vi "HostNoChopper.vi"() -> ()   [LabVIEW 2009]
uses:
  <vilib>/userDefined/High Color/nirio_resource_hc.ctl
  <instrlib>/niScope/Controls/niScope vertical coupling.ctl
  Signal Options.ctl
  Sequence.ctl
  B Field control Signal/B-Generator States.ctl
  <vilib>/Utility/error.llb/DialogType.ctl
  States.ctl
  Raman Measure/Raman.ctl
  Phase Acq.ctl
  <vilib>/DAQmx/write.llb/DAQmx Write (Analog 1D DBL 1Chan NSamp).vi
  <vilib>/DAQmx/configure/trigger.llb/DAQmx Start Trigger (Digital Edge).vi
  <vilib>/DAQmx/configure/timing.llb/DAQmx Timing (Sample Clock).vi
  <vilib>/DAQmx/create/channels.llb/DAQmx Create Channel (AO-Voltage-Basic).vi
  <vilib>/DAQmx/create/channels.llb/DAQmx Create Channel (AI-Voltage-Basic).vi
  <vilib>/DAQmx/read.llb/DAQmx Read (Analog 2D DBL NChan NSamp).vi
  <vilib>/Utility/file.llb/Write To Spreadsheet File (DBL).vi
  <vilib>/rvi/interface/nirviOpenFPGA/nirviOpenFPGA.xnode
  FPGA Bitfiles/MOT2.lvproj_FPGA Target_FPGA-no_chopper.vi.lvbitx
  FPGA-no_chopper.vi
  <vilib>/FPGAPlugInAG/Pxi-7853r/nirviIntfOpen_PXI-7853R.vi
  <vilib>/rvi/interface/nirviReadWriteControl/nirviReadWriteControl.xnode
  <vilib>/LabVIEW Targets/FPGA/Rio/nirio_HostInterface/nirio_ReadBig.vi
  <vilib>/Utility/error.llb/Error Cluster From Error Code.vi
  <vilib>/rvi/errors/niLvFpgaAdjustHostInterfaceError.vi
  <vilib>/rvi/interface/common/niFpgaNodeNameForErrorReporting.ctl
  <vilib>/rvi/errors/niLvFpgaWhatHappensToTopLevelVI.ctl
  <vilib>/RVI Host/nirviSupport.llb/nirviErrorClusterFromErrorCode.vi
  <vilib>/LabVIEW Targets/FPGA/Rio/nirio_HostInterface/nirio_WriteBig.vi
  <vilib>/rvi/interface/nirviCloseFPGA/nirviCloseFPGA.xnode
  <vilib>/FPGAPlugInAG/Pxi-7853r/nirviIntfClose_PXI-7853R.vi
  <vilib>/rvi/interface/nirviMethod/nirviMethod.xnode
  Pulse Acquisition/5122-States.ctl
  <vilib>/Analysis/NI_AALPro.lvlib
  Program Files (x86)/National Instruments/LabVIEW 2009/resource/objmgr/daqmx.rc
  <instrlib>/Agilent ESG Series/Agilent ESG Series.lvlib
  <vilib>/Analysis/NI_AALBase.lvlib
  NiRioSrv.dll
  <instrlib>/niScope/Acquire/Fetch/niScope Fetch.vi
  <instrlib>/niScope/Configure/Trigger/niScope Configure Trigger Edge.vi
  <vilib>/LabVIEW Targets/FPGA/Rio/nirio_HostInterface/nirio_DMAConfigure.vi
  <vilib>/LabVIEW Targets/FPGA/Rio/nirio_HostInterface/nirio_DMAStop.vi
panel:
  in  "Acquisition Delay":dbl[unit] format="%.2f"
  out "Interval Between Samples":dbl[unit]
  out "Actual Sample Rate":dbl[unit]
  in  "Desired Sample Rate":dbl[unit]=100000000.0 caption="Min. Sample Rate" step=1.0 format="%.2p"
  in  "Acquisition Time per Pulse":dbl[unit]=0.0005 format="%#.2g"
  out "Acquisitions Remaining":i32 caption="Number of Runs"
  in  "Number of Pulses to Record":i32=1 caption="Number of Runs" format="%.0p"
  out "Total Acquired Time":dbl[unit]
  out "Total Number of Datapoints":i32=1000000
  out "Total Experiment Time":dbl[unit]
  out "Number of Samples per Pulse":i32
  in  "Vertical range (0 to 10V)":dbl[unit]=4.0 caption="Vertical Range (V)" format="%.2f"
  in  "Vertical coupling":T1=1 caption="Vertical Coupling" items=["AC", "DC", "Ground"]
  in  "Channel":u16(ring) items=["0", "1"]
  out "Phase Frequency Pairs":dbl[][](array[numeric])
  out "Shot Noise File":path
  out "Data Directory":path
  in  "Master Stop":bool
  in  "Tab Control":T2(tab)
  out "Graphing":bool
  in  "Tab Control 3":enum32{"Timing", "TTL Signs"}(tab)
  in  "Trapping (DIO17)":dbl[unit]=0.0015 min=0.0 max=107374.18239999999
  in  "Repump (DIO18)":dbl[unit]=0.0017499999999999998
  in  "Pump (DIO19)":dbl[unit]=0.002
  in  "Memory":bool=TRUE
  in  "Shot Acquisition Trigger Duration":dbl[unit]=9.999999999999999e-06 format="%.2f"
  in  "Shot Acquisition Trigger Delay":dbl[unit] format="%.2f"
  in  "Memory Acquisition Trigger Duration":dbl[unit]=9.999999999999999e-06 format="%.2f"
  in  "Memory Acquisition Trigger Delay":dbl[unit] format="%.2f"
  in  "Acquire Shot":bool=TRUE
  in  "OD Sign":bool=TRUE
  in  "DLCZ Sign":bool=TRUE
  in  "Raman Signal Sign":bool=TRUE
  in  "Raman Control Sign":bool=TRUE
  in  "SPME Gate2 Sign":bool=TRUE
  in  "SPME Gate1 Sign":bool=TRUE
  in  "SPME Signal Sign":bool=TRUE
  in  "SPME Control Sign":bool=TRUE
  in  "Coherent Control Sign":bool
  in  "Coherent Signal Sign":bool
  in  "SQZ AOM Control Sign":bool
  in  "SQZ AOM Signal Sign":bool
  in  "SQZ AOM Signal Delay (DIO6)":dbl[unit]=0.0015
  in  "SQZ AOM Signal Duration (DIO6)":dbl[unit]=0.000125
  in  "Output  Trigger Sign (DIO13)":bool
  out "Measured Acquisition Rate":dbl[unit]=0.02 caption="Acquisition Rate" min=0.0 max=107374.18239999999
  in  "Memory Repetition Period":dbl[unit]=0.025
  out "Measured Memory Sequence Duration":dbl[unit]=0.02 min=0.0 max=107374.18239999999
  in  "DLCZ Period":dbl[unit]=1e-06
  in  "DLCZ Pulse Duration":dbl[unit]=5.0000000000000004e-08
  in  "DLCZ Stop":dbl[unit]=0.004 caption="Stop"
  in  "DLCZ Start":dbl[unit] caption="Start"
  in  "Coherent Signal Delay (DIO6)":dbl[unit]
  in  "Coherent Signal Duration (DIO6)":dbl[unit]=0.000125
  in  "Control Delay(DIO5/1)":dbl[unit] min=0.0 max=107374.18239999999
  in  "Control Duration (DIO5/1)":dbl[unit]=0.000125 min=0.0 max=107374.18239999999
  in  "FPGA Target":T3="FPGA"
  out "Active":bool
  in  "Memory Mode":T4
  out "Generated Signals":digitalwaveform(graph)
  in  "WA Extra 4 (DIO0)":dbl[unit]=0.0003
  in  "WA Extra 4 (DIO0)":dbl[unit]=2.2499999999999998e-05
  in  "WA Extra 3 (DIO0)":dbl[unit]=0.0003225
  in  "WA Extra 3 (DIO0)":dbl[unit]=2.2499999999999998e-05
  in  "WA Extra 2 (DIO0)":dbl[unit]=2.2499999999999998e-05
  in  "WA Extra 2 (DIO0)":dbl[unit]=0.0003
  in  "WA Extra (DIO0)":dbl[unit]=2.2499999999999998e-05
  in  "WA Extra  (DIO0)":dbl[unit]=0.0003225
  in  "WA Extra Sign":bool
  in  "WA Signal Switch 2  (DIO7)":dbl[unit]=0.0005269999999999997
  in  "WA Signal Switch 2 (DIO7)":dbl[unit]=8e-06
  in  "WA Signal Switch Sign":bool=TRUE
  in  "WA Signal Switch (DIO7)":dbl[unit]=0.0003169999999999997
  in  "WA Signal Switch (DIO7)":dbl[unit]=8e-06
  in  "WA Repetition Period":dbl[unit]=0.0075
  in  "WA ControlS Sign":bool=TRUE
  in  "WA Output  Trigger  Sign (DIO1)":bool
  in  "WA Signal Sign":bool
  in  "WA Repump Sign":bool
  in  "WA Pump Sign":bool
  in  "WA Control Sign":bool=TRUE
  in  "WA ControlS 2 (DIO6)":dbl[unit]=5.999999999999999e-06
  in  "WA ControlS 2 (DIO6)":dbl[unit]=0.0005249999999999996
  in  "WA Control Switch 1(DIO6)":dbl[unit]=0.00031499999999999963 min=0.0 max=107374.18239999999
  in  "WA Control Switch 1 (DIO6)":dbl[unit]=5.999999999999999e-06 min=0.0 max=107374.18239999999
  in  "WA Signal (DIO5)":dbl[unit]=2.2499999999999998e-05
  in  "WA Signal (DIO5)":dbl[unit]=0.0003
  in  "WA Repump (DIO3)":dbl[unit]=0.0007
  in  "WA Repump (DIO3)":dbl[unit]
  in  "WA Pump (DIO2)":dbl[unit]=0.0007
  in  "WA Pump (DIO2)":dbl[unit]
  in  "WA Control 2 (DIO4)":dbl[unit]=1.9999999999999998e-05
  in  "WA Control 2 (DIO4)":dbl[unit]=0.0005124999999999995
  in  "WA Control 1 (DIO4)":dbl[unit]=0.0003024999999999995 min=0.0 max=107374.18239999999
  in  "WA Control 1 (DIO4)":dbl[unit]=1.9999999999999998e-05 min=0.0 max=107374.18239999999
  out "WA Active":bool
  out "WA Reset Interval (test)":u64
  in  "Activate Raman Acquisition":bool
  in  "Scan Frequency":bool
  out "Measurement":dbl[][](graph) caption="Pulse Monitor"
  out "Raman Measure - Frequency Scan":cluster{dbl[], dbl[]}[](graph)
  in  "Ramand Control Duration (DIO5)":dbl[unit]=0.000125 min=0.0 max=107374.18239999999
  in  "Raman Control Delay(DIO5)":dbl[unit] min=0.0 max=107374.18239999999
  in  "Raman Signal Delay (DIO6)":dbl[unit]=4.9999999999999996e-05
  in  "Raman Signal Duration (DIO6)":dbl[unit]=0.000125
  in  "Linewidth":dbl[unit]=5234000.0
  in  "Detuning":dbl[unit]=10000000.0
  out "Optical Density Chart":T5(graph)
  in  "Tab Control 2":T6(tab)=enum."Threshold Settings"
  out "Optical Density Signal 2":string
  out "Optical Density Signal 1":string
  in  "OD Acquisition Delay":dbl[unit] format="%.2f"
  out "Acquisition Count":i32
  in  "Number of Measurements":u32=10
  in  "Samples per Channel":i32=2048 caption="Measurement Samples"
  out "Current Frequency":dbl[unit]
  in  "Start Frequency":dbl[unit]=-5000000.0
  in  "Stop Frequency":dbl[unit]=5000000.0
  in  "Resonance Frequency":dbl[unit]=100000000.0
  in  "Number of Frequency Intervals":u32=100
  out "Frequency Interval":dbl[unit]
  in  "Signal 2 Gain":dbl=1.0
  in  "Signal 2 Offset":dbl[unit]
  in  "Signal 1 Gain 2":dbl=1.0
  in  "Signal 1 Offset":dbl[unit]
  in  "Show Signal 2":bool
  in  "Show Reference":bool=TRUE
  in  "Show Signal 1":bool
  in  "Lower Threshold (% of Min)":dbl=110.0
  in  "Upper Threshold (% of Max)":dbl=95.0
  in  "Trigger source":tag="/Julien/PFI2"
  in  "Input Channels":tag="Julien/ai0:2"
  in  "VISA session":refnum<visa-resource-name>="GPIB0::19::INSTR"
  in  "Minimum Value":dbl[unit]=-10.0
  in  "Maximum Voltage":dbl[unit]=10.0
  in  "Acquisition Rate":dbl[unit]=5000000.0
  out "Raman Measurement File Root":path
  out "Raman Measurement File":path
  in  "Opt Density Delay (DIO7)":dbl[unit]
  in  "Opt Density Duration (DIO7)":dbl[unit]=9.999999999999999e-06
  in  "SPME Start":dbl[unit]
  in  "SPME Signal Delay(DIO5/1)":dbl[unit] min=0.0 max=107374.18239999999
  in  "SPME Signal Duration (DIO5/1)":dbl[unit]=0.000125 min=0.0 max=107374.18239999999
  in  "SPME Control Delay(DIO5/1)":dbl[unit] min=0.0 max=107374.18239999999
  in  "SPME Control Duration (DIO5/1)":dbl[unit]=0.000125 min=0.0 max=107374.18239999999
  in  "Num of SPME Pulses per Mem Seq":u64=100
  in  "SPME Period":dbl[unit]
  in  "SPME Leakage Gate Delay":dbl[unit]
  in  "SPME Leakage Gate Duration":dbl[unit]
  in  "SPME Signal Gate Delay":dbl[unit]
  in  "SPME Signal Gate Duration":dbl[unit]
  out "N1":u64
  out "N2":u64
  out "Number of Trials":u64
  in  "Desired Number of Trials":u64=100000
  in  "Tab Control 4":enum32{"Page 1", "Acquisition Settings"}(tab)=enum."Acquisition Settings"
  out "Quadrature Pulses File":path
  out "Reference Pulse File":path
  out "Acquisition Sequence":dbl[][](graph)
  in  "Get Reference Parameters":bool
  in  "Capture":bool
  in  "Acquire Data":bool
  out "Global EIT Delay":dbl[unit] format="%#.2g"
  out "Writing Phase to File":bool
  in  "Acquire Phase":bool
  in  "Physical Channel":tag="Julien/ai0,Julien/ai3"
  in  "Phase Acquisition Rate":dbl[unit]=5000000.0 caption="Sample Rate" format="%0.2f"
  in  "Minimum Value":dbl=-0.5 format="%0.2f"
  in  "Maximum Value":dbl=0.5 format="%0.2f"
  in  "samples per channel":i32=130000
  in  "Trigger Source 2":tag="/Julien/PFI1"
  out "Phase Acquisition Sampling Freq":dbl
  in  "Phase Extraction":T7(tab)=enum."Fourrier Transform Filtering Settings"
  out "Phase Monitor":dbl[][](graph)
  out "Raw Phase, Trigger, Extracted Phase Data":path
  out "Phase-Frequency Pairs":path
  out "Normalized Envelope":waveform(dbl)(graph)
  out "detected frequency":dbl format="%.4p"
  in  "Low Pass Filter Cutoff Freq: Hz":dbl=200.0
  in  "Filter Order":i32=1 min=1 max=10 step=1
  out "Memory Duration":dbl[unit]
  in  "Global Delay":dbl[unit]=3e-06
  in  "High Voltage (V Hi)":dbl[unit]=5.0
  in  "Trigger Control":bool=TRUE
  in  "Activate B-Field":bool=TRUE
  out "B-Field Control Signal":dbl[](graph)
  in  "V4":dbl[unit]
  in  "V3":dbl[unit]
  in  "V2":dbl[unit]=-5.0
  in  "V1":dbl[unit]=-5.0 min=-10.0 max=10.0
  in  "B":dbl[unit]=0.0046
  in  "A":dbl[unit]=0.0007
  in  "Trigger Source":tag="/Julien/PFI0"
  in  "Output Channel":tag="Julien/ao0"
  out "Risetime Chart":cluster{dbl}(graph)
  out "Falltime Chart":cluster{dbl}(graph)
  out "Width Chart":cluster{dbl}(graph)
  out "Delay Chart":cluster{dbl}(graph)
  out "Amplitude Chart":cluster{dbl}(graph)
  out "Risetime":string
  out "Falltime":string
  out "Pulse Width":string
  out "Delay":string
  out "Amplitude":string
  out "Current State":T8
  out "Cut Initiated":dbl[unit]
  out "Memory Mode 2":T4=enum."Coherent Memory Sequence"
  out "Memory Timer":dbl[unit]
  out "Global Time":dbl[unit]
  out "Last DLCZ Period":dbl[unit]
  out "Raman/OD Aquisition Delay":dbl[unit]
  out "Last SPME Interval Between Resets":dbl[unit]
  out "SPME Count":u64
  out "Read SPME Signal Stop":dbl[unit]
  out "Read SPME Period":dbl[unit]
  out "Read SPME Signal Start":dbl[unit]
  out "Read Num of SPME Pulses per Mem Seq":u64=100
  out "Read SPME Control Start":dbl[unit]
  out "Read SPME Control Stop":dbl[unit]
  out "Read SPME Start":dbl[unit]
  out "Memory Acquisition Trigger Delay":dbl[unit]
  out "Reference Pulse":dbl[](array[numeric])
  out "Channel String":string
  # "Delays"
  # "Durations"
  # "Coherent Signal (DIO21)"
  # "Period"
  # "Chopper Measurement and MOT Timing"
  # "Extinction Time"
  # "Alignment - Lights On"
  # "SQZ Signal (DIO23)"
  # "DLCZ Pulse Train (Signal - DIO21)"
  # "Width"
  # "Control  (DIO20)"
  # "Delays"
  # "Durations"
  # "signs"
  # "Delays"
  # "Durations"
  # "Raman Signal (DIO21)"
  # "Raman Control (DIO20"
  # "Offset"
  # "Gain"
  # "Signal 1"
  # "Signal 2"
  # "File Format:   Freq   OD1   OD2"
  # "Optical Density (DIO22)"
  # "Delay"
  # "Duration"
  # "SPME Control  (DIO20)"
  # "SPME Signal  (DIO21)"
  # "SPME Leakage Gate"
  # "SPME Signal Gate"
  # "SPME Debug"
  # "Optical Pulse Acquisition"
  # "Example Diagram"
  # "Voltages"
  # "Intervals"
  # "Trigger must be sent \nto begin generation"
  # "Pulse Statistics"
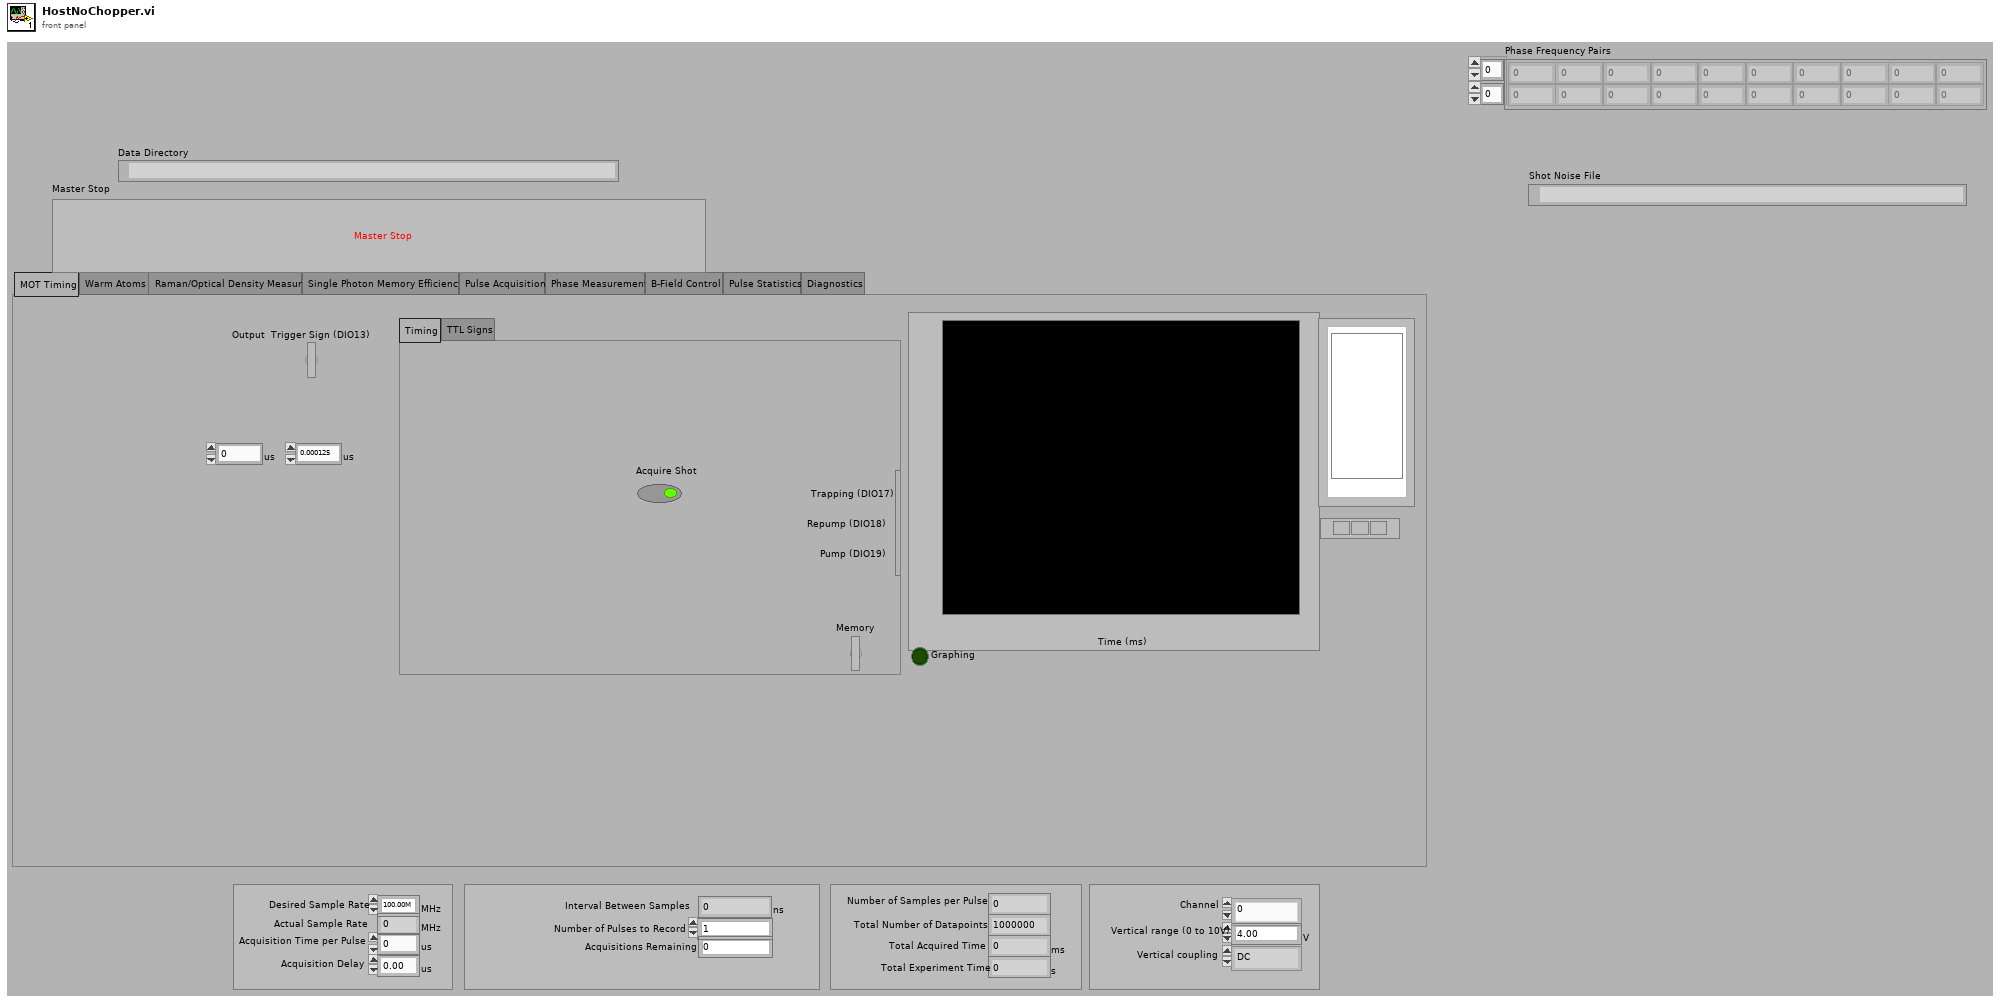
[diagram p1: front panel]
types:
  T1 = typedef "niScope vertical coupling.ctl" = i32
  T2 = enum32{"MOT Timing", "Warm Atoms", "Raman/Optical Density Measure", "Single Photon Memory Efficiency", "Pulse Acquisition", "Phase Measurement", "B-Field Control", "Pulse Statistics", "Diagnostics"}
  T3 = typedef "nirio_resource_hc.ctl" = tag
  T4 = typedef "Signal Options.ctl" = enum16{"Cycle Trap - Standby", "Generate DLCZ Pulses", "Measure Optical Density", "Measure Raman", "Single Photon Memory Efficiency", "Coherent Memory Sequence", "Squeezed AOM Memory Sequence", "Squeezed Chopper Memory Sequence"}
  T5 = cluster{"Optical Density 1":dbl, "Optical Density 2":dbl}
  T6 = enum32{"Parameters", "Threshold Settings", "Acquisition Settings"}
  T7 = enum32{"Arches and Phase Monitor", "Fourrier Transform Filtering Settings"}
  T8 = typedef "Sequence.ctl" = enum16{"Build MOT", "Memory Sequence", "Alignment - Lights On"}
  T9 = enum16{"open", "replace", "create", "open or create", "replace or create", "replace or create with confirmation"}
  T10 = typedef "Phase Acq.ctl" = enum16{"Start Phase Acquisition", "Monitor Phase", "Stop Phase Acquisition", "Restart", "Standby"}
  T11 = typedef "Raman.ctl" = enum16{"Initialize", "Monitor Pulses", "Stop Raman Acquisition", "Scan Frequency", "Output Data", "Standby"}
  T12 = typedef "States.ctl" = enum16{"Initialize", "Send Data", "Receive Data", "Update Graph", "Check for Activity", "Close"}
  T13 = typedef "DialogType.ctl" = u16
  T14 = typedef "B-Generator States.ctl" = enum16{"Initialize", "Start Task", "Check Task", "Stop Task", "Stop"}
  T15 = typedef "5122-States.ctl" = enum16{"Initialize Card", "Continuous Mode", "Fetch", "Snapshot Acquistion", "Standby", "Record DataFile", "Exit"}
  T16 = cluster{"Optical Density 1":dbl, "Optical Density 2":dbl}[]
  T17 = cluster{"Phase Acquisition Sampling Freq":dbl, "samples per channel":i32}
  T18 = typedef "niFpgaNodeNameForErrorReporting.ctl" = enum16{"Open FPGA VI Reference", "Read/Write Control", "Invoke Method: Abort", "Invoke Method: Acknowledge IRQ", "Invoke Method: Download", "Invoke Method: FIFO.Configure", "Invoke Method: FIFO.Read", "Invoke Method: FIFO.Start", "Invoke Method: FIFO.Stop", "Invoke Method: FIFO.Write", "Invoke Method: Reset", "Invoke Method: Run", "Invoke Method: Wait on IRQ", "Close FPGA VI Reference"}
  T19 = typedef "niLvFpgaWhatHappensToTopLevelVI.ctl" = enum16{"top level VI scripted behind XNode", "top level VI inlined behind XNode"}
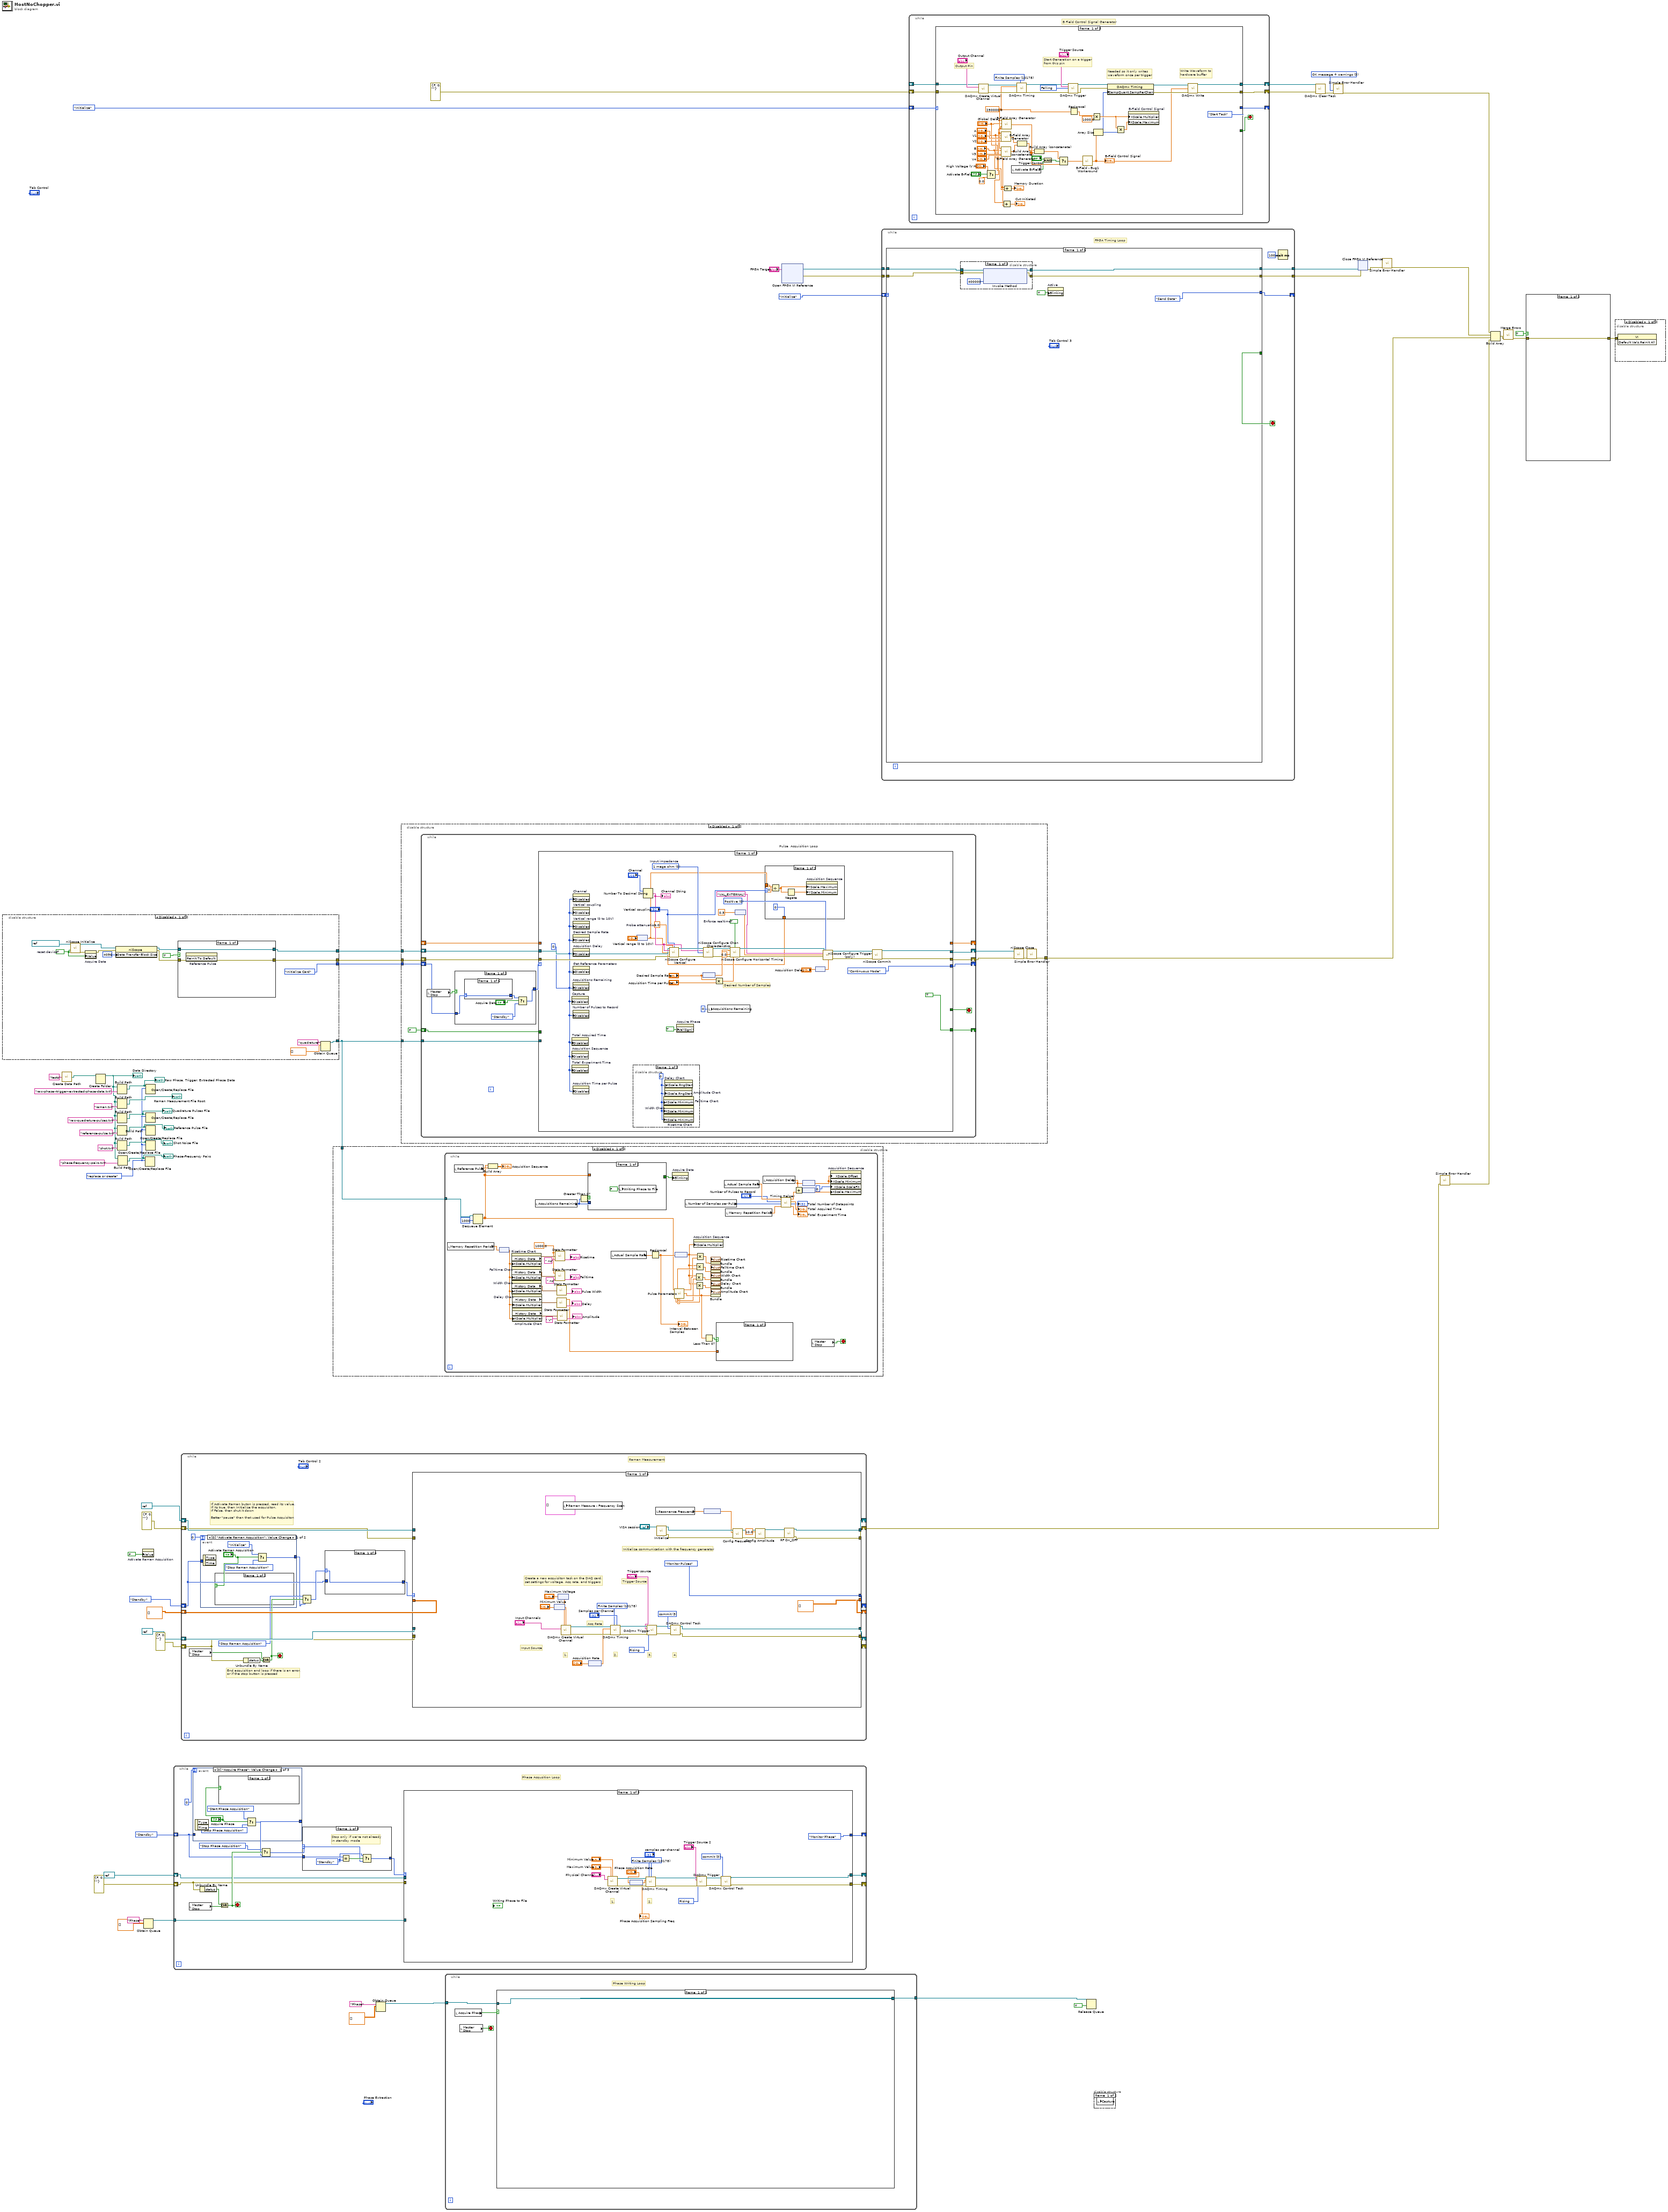
[diagram p0: block diagram]
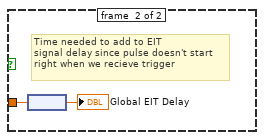
[diagram p2: hidden frame]
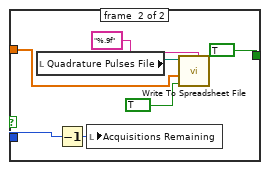
[diagram p3: hidden frame]
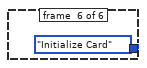
[diagram p9: hidden frame]
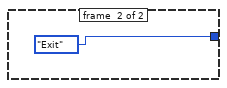
[diagram p10: hidden frame]
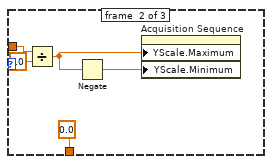
[diagram p12: hidden frame]
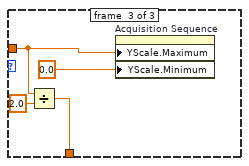
[diagram p13: hidden frame]
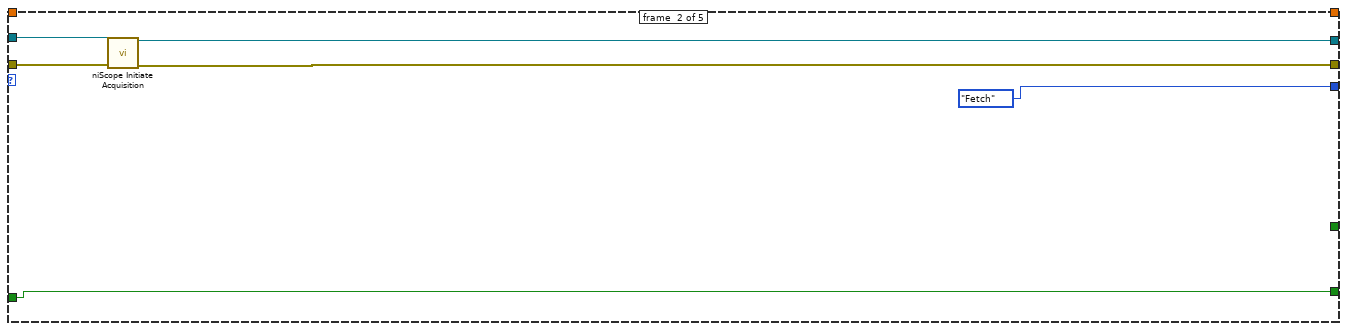
[diagram p14: hidden frame]
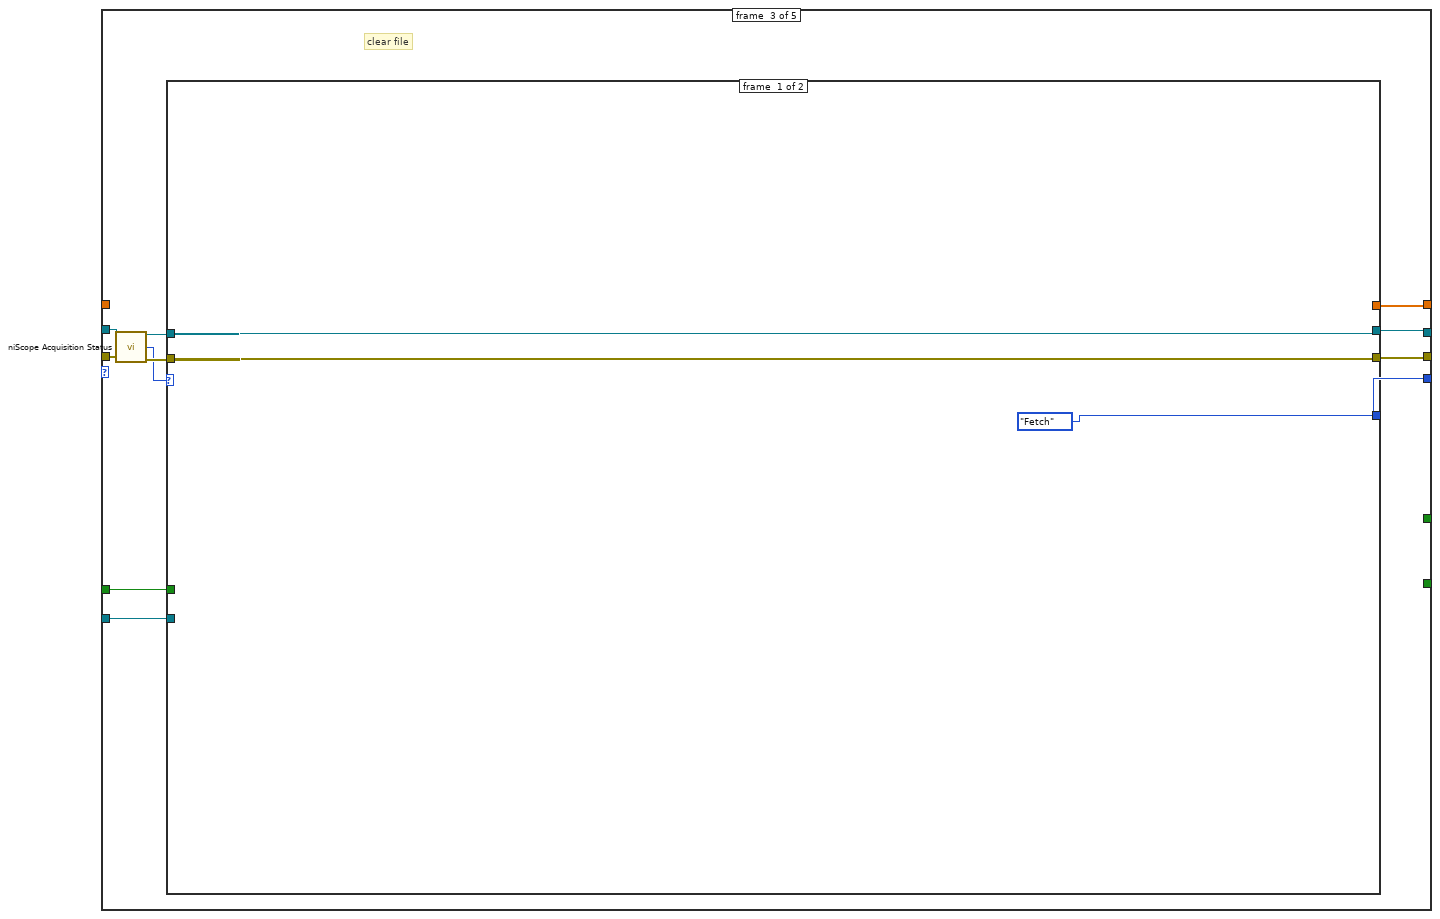
[diagram p15: hidden frame]
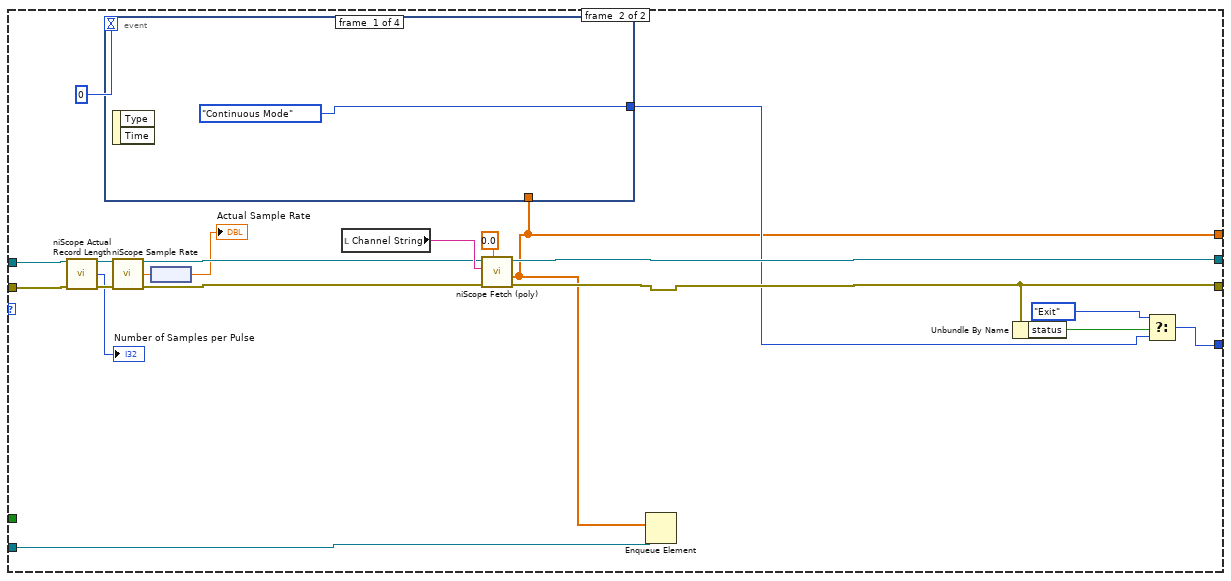
[diagram p16: hidden frame]
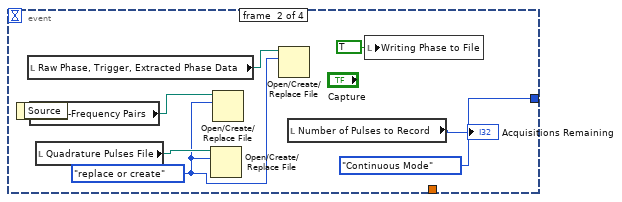
[diagram p17: hidden frame]
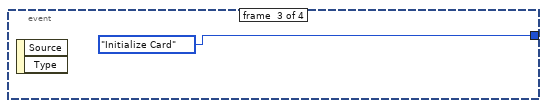
[diagram p18: hidden frame]
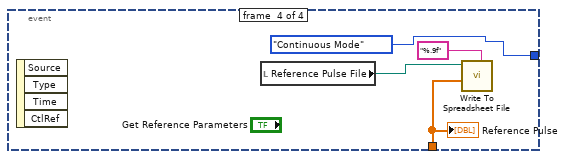
[diagram p19: hidden frame]
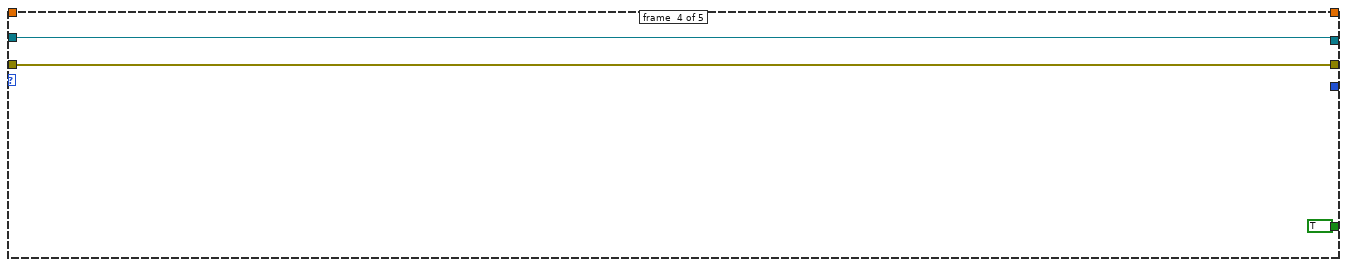
[diagram p20: hidden frame]
diagram:
  w2 = T9."replace or create" ("operation (0:open)")
  w57 = T13 3 items=["no dialog", "OK message", "continue or stop message", "OK message + warnings", "continue/stop + warnings"] ("type of dialog (OK msg:1)")
  n1 = disable-structure shown="Disabled" {
    disable-tunnel: [w67 _] -> w60
    disable-tunnel: [w65 _] -> w59
    disable-tunnel: [5122-States."Initialize Card" ("Enum") _] -> w58
    disable-tunnel: [w61 _] -> w1
    frame #0 {
      w70 = TRUE  # reset device
      n2 = call <instrlib>:"niScope Initialize.vi"("resource name"=refnum<k15> "Acquisition" ("Resource name 5"), "reset device"=w70) -> ("instrument handle"=w74:refnum<k15>, "error out"=w72:errorcluster)  [unwired: 2 in, 10 out]
      n3 = property on="Acquire Data" class="Bool (strict)"(error in=w72, "Value"=w70) -> (error out=w71:errorcluster)  [unwired: 1 in, 1 out]
      n4 = property class="niScope"(reference=w74, error in=w71, "Data Transfer Block Size"=4096) -> (reference out=w68:refnum<k15>, error out=w66:errorcluster)
      n5 = case shown="True" TRUE {
        tunnel: [w77 w79] -> w67
        tunnel: w68 -> [w77 w79]
        tunnel: [w76 w78] -> w65
        tunnel: w66 -> [w76 w78]
        frame #0 {
          n6 = invoke on="Reference Pulse" class="Arr (strict)" method="Reinit To Default"() -> ()  [unwired: 3 in, 3 out]
        }
        frame #1 {
        }
      }
      n7 = Obtain Queue(name (unnamed)="quadrature", element data type=dbl[] [] ("wfm")) -> (queue out=w61:refnum<queue>)  [unwired: 3 in, 2 out]
    }
    frame #1 {
    }
  }
  n8 = call "Create Data Path.vi"("Data Directory Name"="tests") -> ("appended path"=w13:path)
  n9 = Create Folder(path (use dialog)=w13) -> (created path=w4:path)  [unwired: 2 in, 2 out]
  "Data Directory" <- w4
  n10 = Build Path(base path=w4, name or relative path="raw-phase--trigger--extracted-phase-data.txt") -> (appended path=w11:path)
  "Raw Phase, Trigger, Extracted Phase Data" <- w11
  n11 = Build Path(base path=w4, name or relative path="raman.txt") -> (appended path=→"Raman Measurement File Root":path)
  n12 = Build Path(base path=w4, name or relative path="raw-quadrature-pulses.txt") -> (appended path=w9:path)
  "Quadrature Pulses File" <- w9
  n13 = Build Path(base path=w4, name or relative path="reference-pulse.txt") -> (appended path=w8:path)
  "Reference Pulse File" <- w8
  n14 = Build Path(base path=w4, name or relative path="shot.txt") -> (appended path=w7:path)
  "Shot Noise File" <- w7
  n15 = Build Path(base path=w4, name or relative path="phase-frequency-pairs.txt") -> (appended path=w3:path)
  "Phase-Frequency Pairs" <- w3
  n16 = property on="Activate Raman Acquisition" class="Bool (strict)"("Value"=FALSE ("Activate Raman Acquisition")) -> ()  [unwired: 2 in, 2 out]
  n17 = Obtain Queue(name (unnamed)="Phase", element data type=dbl[][] [] ("data")) -> (queue out=w22:refnum<queue>)  [unwired: 3 in, 2 out]
  n18 = Open/Create/Replace File(file path (use dialog)=w3, operation (0:open)=w2) -> ()  [unwired: 4 in, 3 out]
  n19 = Open/Create/Replace File(file path (use dialog)=w11, operation (0:open)=w2) -> ()  [unwired: 4 in, 3 out]
  n20 = Open/Create/Replace File(file path (use dialog)=w9, operation (0:open)=w2) -> ()  [unwired: 4 in, 3 out]
  n21 = Open/Create/Replace File(file path (use dialog)=w8, operation (0:open)=w2) -> ()  [unwired: 4 in, 3 out]
  n22 = Open/Create/Replace File(file path (use dialog)=w7, operation (0:open)=w2) -> ()  [unwired: 4 in, 3 out]
  n23 = while {
    shift-right: [w86] -> _
    shift-left: refnum<k21> refnum ("task out") -> [w84]
    shift-right: [w85] -> _
    shift-left: errorcluster {"status"=FALSE, "code"=0, "source"=""} ("error out") -> [w82]
    shift-right: [w83] -> _
    shift-left: Phase_Acq."Standby" ("Enum") -> [w88]
    tunnel: w22 -> [w80]
    stop <- w91 stop-if-true
    # "Phase Acqusition Loop"
    n24 = local read "Master Stop"() -> (w93:bool)
    n25 = event shown="[0] \"Acquire Phase\": Value Change" {
      selector: _ -> [_ _ _]
      dyn-events: _ -> [_ _ _]
      timeout: 0 -> [_ _ _]
      tunnel: [w158 Phase_Acq."Restart" ("Enum") w161] -> w90
      tunnel: w88 -> [_ _ w161]
      event #0 {
        n26 = event-data() -> ()  [unwired: 1 in, 2 out]
        n27 = case shown="True" "Acquire Phase" {
          frame #0 {
          }
          frame #1 {
            # "Disabled Raman Acquisiton if we want to start\nPhase Acq.  Uses same cards"
            n28 = property on="Activate Raman Acquisition" class="Bool (strict)"("Val(Sgnl)"=FALSE ("Value (Signaling)")) -> ()  [unwired: 2 in, 2 out]
          }
        }
        n29 = Select(t=Phase_Acq."Start Phase Acquisition" ("Enum"), s="Acquire Phase", f=Phase_Acq."Stop Phase Acquisition" ("Enum")) -> (s? t:f=w158:T10)
      }
      event #1 {
        n30 = event-data() -> ()  [unwired: 1 in, 3 out]
      }
      event #2 {
        n31 = event-data() -> ()  [unwired: 1 in, 2 out]
      }
    }
    n32 = Unbundle By Name(w82) -> ("status"=w81:bool)
    n33 = Or(x=w81, y=w93) -> (x .or. y?=w91:bool)
    n34 = Select(t=Phase_Acq."Stop Phase Acquisition" ("Enum"), s=w91, f=w90) -> (s? t:f=w92:T10)
    n35 = case shown="\"Standby\"" w92 {
      selector: w92 -> [w148 w151 w152 w153 w154]
      tunnel: w88 -> [w150 _ _ _ _]
      tunnel: [w147 w151 w152 w153 w154] -> w87
      frame #0 {
        w146 = Phase_Acq."Standby" ("Enum")
        # "Stop only if we're not already\nin standby mode"
        n36 = Equal?(x=w150, y=w146) -> (x = y?=w149:bool)
        n37 = Select(t=w146, s=w149, f=w148) -> (s? t:f=w147:T10)
      }
      frame #1 {
      }
      frame #2 {
      }
      frame #3 {
      }
      frame #4 {
      }
    }
    n38 = case shown="\"Restart\"" w87 {
      tunnel: [w98 refnum<k21> refnum ("task out") refnum<k21> refnum ("task out") refnum<k21> refnum ("task out") w145] -> w86
      tunnel: [w97 errorcluster {"status"=FALSE, "code"=0, "source"=""} ("error out") errorcluster {"status"=FALSE, "code"=0, "source"=""} ("error out") errorcluster {"status"=FALSE, "code"=0, "source"=""} ("error out") w144] -> w85
      tunnel: w84 -> [_ w118 w125 _ w143]
      tunnel: w82 -> [_ w117 w124 _ w142]
      tunnel: [Phase_Acq."Monitor Phase" ("Enum") Phase_Acq."Standby" ("Enum") Phase_Acq."Start Phase Acquisition" ("Enum") Phase_Acq."Standby" ("Enum") Phase_Acq."Monitor Phase" ("Enum")] -> w83
      tunnel: w80 -> [_ _ _ _ w131]
      frame #0 {
        w99 = 3 items=["verify"=2, "reserve"=4, "commit"=3, "unreserve"=5, "abort"=6] ("action")
        w103 = 10280 items=["Rising"=10280, "Falling"=10171] ("edge")
        w113 = 10178 items=["Finite Samples"=10178, "Continuous Samples"=10123] ("sample mode")
        # "2."
        # "1."
        n39 = call-poly <vilib>:"DAQmx Create Virtual Channel.vi"("maximum value"="Maximum Value", "minimum value"="Minimum Value", "physical channels"="Physical Channel") -> ("task out"=w111:refnum<k21>, "error out"=w110:errorcluster)  [unwired: 6 in, 5 out]
        n40 = node("Phase Acquisition Rate") -> (w95:dbl)
        "Phase Acquisition Sampling Freq" <- w95
        n41 = call-poly <vilib>:"DAQmx Timing.vi"("task/channels in"=w111, "sample mode"=w113, "samples per channel"="samples per channel", "rate"=w95, "error in"=w110) -> ("task out"=w105:refnum<k21>, "error out"=w104:errorcluster)  [unwired: 2 in, 7 out]
        n42 = call-poly <vilib>:"DAQmx Trigger.vi"("task/channels in"=w105, "source"="Trigger Source 2", "edge"=w103, "error in"=w104) -> ("task out"=w101:refnum<k21>, "error out"=w100:errorcluster)  [unwired: 10 in]
        n43 = call <vilib>:"DAQmx Control Task.vi"("task/channels in"=w101, "action"=w99, "error in"=w100) -> ("task out"=w98:refnum<k21>, "error out"=w97:errorcluster)  [unwired: 11 in]
      }
      frame #1 {
        w120 = T13 3 items=["no dialog", "OK message", "continue or stop message", "OK message + warnings", "continue/stop + warnings"] ("type of dialog (OK msg:1)")
        n44 = call <vilib>:"DAQmx Clear Task.vi"("task in"=w118, "error in"=w117) -> ("error out"=w119:errorcluster)  [unwired: 13 out]
        n45 = call <vilib>:"Simple Error Handler.vi"("type of dialog (OK msg:1)"=w120, "error in (no error)"=w119) -> ()  [unwired: 8 out]
      }
      frame #2 {
        w127 = T13 3 items=["no dialog", "OK message", "continue or stop message", "OK message + warnings", "continue/stop + warnings"] ("type of dialog (OK msg:1)")
        n46 = call <vilib>:"DAQmx Clear Task.vi"("task in"=w125, "error in"=w124) -> ("error out"=w126:errorcluster)  [unwired: 13 out]
        n47 = call <vilib>:"Simple Error Handler.vi"("type of dialog (OK msg:1)"=w127, "error in (no error)"=w126) -> ()  [unwired: 8 out]
      }
      frame #3 {
      }
      frame #4 {
        w133 = u8 0 ("X Scale.Scale Fit")
        # "4."
        n48 = local read "Phase Acquisition Rate"() -> (w140:dbl[unit])
        n49 = local read "samples per channel"() -> (w137:i32)
        n50 = node(w140) -> (w139:dbl)
        n51 = Reciprocal(x=w139) -> (1/x=w136:dbl)
        n52 = Multiply(x=w137, y=w136) -> (x*y=w135:dbl)
        n53 = Add(x=w133, y=w135) -> (x+y=w134:dbl)
        n54 = property on="Phase Monitor" class="WFGraph (strict)"("XScale.Offset"=w133, "XScale.Minimum"=w133, "XScale.Maximum"=w134, "XScale.ScaleFit"=u8 0 ("X Scale.Scale Fit"), "XScale.Multiplier"=w136) -> ()  [unwired: 2 in, 2 out]
        n55 = call-poly <vilib>:"DAQmx Read.vi"("task/channels in"=w143, "error in"=w142) -> ("task out"=w145:refnum<k21>, "data"=w132:dbl[][], "error out"=w144:errorcluster)  [unwired: 2 in, 9 out]
        n56 = Enqueue Element(queue=w131, element=w132) -> ()  [unwired: 2 in, 3 out]
      }
    }
  }
  n57 = while {
    shift-right: [w177] -> _
    shift-left: Raman."Standby" ("Raman State") -> [w163]
    shift-right: [w180] -> _
    shift-left: refnum<k21> refnum ("task out") -> [w176]
    shift-right: [w181] -> _
    shift-left: errorcluster {"status"=FALSE, "code"=0, "source"=""} ("error out") -> [w171]
    shift-right: [w172] -> _
    shift-left: dbl[][] [] -> [w175]
    shift-right: [w178] -> _
    shift-left: refnum<visa-resource-name> refnum ("VISA Resource Name Out") -> [w174]
    shift-right: [w179] -> w36
    shift-left: errorcluster {"status"=FALSE, "code"=0, "source"=""} ("error out") -> [w173]
    stop <- w167 stop-if-true
    # "If Activate Raman buton is pressed, read its value.\nIf its true, then Initialize the acquisiton, \nIf False, then shut it down\n\nBetter \"pause\" than that used for Pulse Acquisiton"
    # "End acquisition and loop if there is an error, \nor if the stop button is pressed"
    # "Raman Measurement"
    n58 = local read "Master Stop"() -> (w169:bool)
    n59 = event shown="[0] \"Activate Raman Acquisition\": Value Change" {
      selector: _ -> [_ _]
      dyn-events: _ -> [_ _]
      timeout: 0 -> [_ _]
      tunnel: [w193 w197] -> w165
      tunnel: w163 -> [_ w197]
      event #0 {
        n60 = event-data() -> ()  [unwired: 1 in, 2 out]
        n61 = case shown="True" "Activate Raman Acquisition" {
          frame #0 {
          }
          frame #1 {
            # "Disabled Phase Acquisiton if we want to start\nRaman Acq.  Uses same cards"
            n62 = property on="Acquire Phase" class="Bool (strict)"("Val(Sgnl)"=FALSE ("Value (Signaling)")) -> ()  [unwired: 2 in, 2 out]
          }
        }
        n63 = Select(t=Raman."Initialize" ("Raman State"), s="Activate Raman Acquisition", f=Raman."Stop Raman Acquisition" ("Raman State")) -> (s? t:f=w193:T11)
      }
      event #1 {
        n64 = event-data() -> ()  [unwired: 1 in, 2 out]
      }
    }
    n65 = Unbundle By Name(w171) -> ("status"=w170:bool)
    n66 = Or(x=w169, y=w170) -> (x .or. y?=w167:bool)
    n67 = Select(t=Raman."Stop Raman Acquisition" ("Raman State"), s=w167, f=w165) -> (s? t:f=w164:T11)
    n68 = case shown="\"Standby\"" w164 {
      selector: w164 -> [w182 w183 w185 w189 w190 w191]
      tunnel: w163 -> [_ _ w188 _ _ _]
      tunnel: [w182 w183 w184 w189 w190 w191] -> w162
      frame #0 {
      }
      frame #1 {
      }
      frame #2 {
        w186 = Raman."Standby" ("Raman State")
        # "Stop only if we're not already\nin standby mode"
        n69 = Equal?(x=w188, y=w186) -> (x = y?=w187:bool)
        n70 = Select(t=w186, s=w187, f=w185) -> (s? t:f=w184:T11)
      }
      frame #3 {
      }
      frame #4 {
      }
      frame #5 {
      }
    }
    n71 = case shown="\"Monitor Pulses\"" w162 {
      tunnel: [w216 w272 w308 w359 errorcluster {"status"=FALSE, "code"=0, "source"=""} ("error out") w382] -> w181
      tunnel: [w217 w273 w307 w360 refnum<k21> refnum ("task out") refnum<k21> refnum ("task out")] -> w180
      tunnel: [w204 w277 w293 w357 w368 errorcluster {"status"=FALSE, "code"=0, "source"=""} ("error out")] -> w179
      tunnel: [w203 w278 w294 w358 w369 refnum<visa-resource-name> refnum ("VISA Resource Name Out")] -> w178
      tunnel: [Raman."Monitor Pulses" ("Raman State") w271 Raman."Output Data" ("Raman State") Raman."Monitor Pulses" ("Raman State") Raman."Standby" ("Raman State") Raman."Standby" ("Raman State")] -> w177
      tunnel: w176 -> [_ w275 w300 w360 _ w384]
      tunnel: w171 -> [_ w274 w299 w359 _ w383]
      tunnel: w175 -> [_ _ _ w362 _ _]
      tunnel: w174 -> [_ w278 w297 w358 w369 w372]
      tunnel: w173 -> [_ w277 w296 w357 w368 w371]
      tunnel: [dbl[][] [] ("Frequency/Delta Pairs") _ w284 _ _ _] -> w172
      frame #0 {
        w232 = 10280 items=["Rising"=10280, "Falling"=10171] ("edge")
        w223 = 3 items=["verify"=2, "reserve"=4, "commit"=3, "unreserve"=5, "abort"=6] ("action")
        w224 = 10178 items=["Finite Samples"=10178, "Continuous Samples"=10123] ("sample mode")
        # "Initialize communication with the frequency generator"
        # "Create a new acquisiton task on the DAQ card, \nset settings for voltage, Acq rate, and triggers"
        # "Input Source"
        # "Acq Rate"
        # "Trigger Source"
        # "4."
        # "3."
        # "2."
        # "1."
        n72 = node("Minimum Value") -> (w198:dbl)
        n73 = node("Maximum Voltage") -> (w199:dbl)
        n74 = call-poly <vilib>:"DAQmx Create Virtual Channel.vi"("maximum value"=w199, "minimum value"=w198, "physical channels"="Input Channels") -> ("task out"=w226:refnum<k21>, "error out"=w229:errorcluster)  [unwired: 11 in]
        n75 = local write "Raman Measure - Frequency Scan"(cluster{dbl[], dbl[]}[] [] ("Raman Measure")) -> ()
        n76 = node("Acquisition Rate") -> (w200:dbl)
        n77 = call-poly <vilib>:"DAQmx Timing.vi"("task/channels in"=w226, "sample mode"=w224, "samples per channel"="Samples per Channel", "rate"=w200, "error in"=w229) -> ("task out"=w222:refnum<k21>, "error out"=w221:errorcluster)  [unwired: 9 in]
        n78 = call-poly <vilib>:"DAQmx Trigger.vi"("task/channels in"=w222, "source"="Trigger source", "edge"=w232, "error in"=w221) -> ("task out"=w220:refnum<k21>, "error out"=w219:errorcluster)  [unwired: 10 in]
        n79 = local read "Resonance Frequency"() -> (w211:dbl[unit])
        n80 = call <instrlib>:"Initialize.vi"("VISA Resource Name"="VISA session") -> ("VISA Resource Name Out"=w213:refnum<visa-resource-name>, "error out"=w212:errorcluster)  [unwired: 4 in, 9 out]
        n81 = call <vilib>:"DAQmx Control Task.vi"("task/channels in"=w220, "action"=w223, "error in"=w219) -> ("task out"=w217:refnum<k21>, "error out"=w216:errorcluster)  [unwired: 11 in]
        n82 = node(w211) -> (w210:dbl)
        n83 = call <instrlib>:"Config Frequency.vi"("VISA Resource Name"=w213, "Frequency (1000.0)"=w210, "error in (no error)"=w212) -> ("VISA Resource Name Out"=w209:refnum<visa-resource-name>, "error out"=w208:errorcluster)  [unwired: 6 in, 5 out]
        n84 = call <instrlib>:"Config Amplitude.vi"("VISA Resource Name"=w209, "Amplitude (-135.00)"=10.0, "error in (no error)"=w208) -> ("VISA Resource Name Out"=w206:refnum<visa-resource-name>, "error out"=w205:errorcluster)  [unwired: 5 in, 6 out]
        n85 = call <instrlib>:"RF On_OFF.vi"("VISA Resource Name"=w206, "error in (no error)"=w205) -> ("VISA Resource Name Out"=w203:refnum<visa-resource-name>, "error out"=w204:errorcluster)  [unwired: 1 in, 11 out]
      }
      frame #1 {
        n86 = local read "Acquisition Rate"() -> (w258:dbl[unit])
        n87 = local read "OD Acquisition Delay"() -> (w257:dbl[unit])
        n88 = local read "Samples per Channel"() -> (w259:i32)
        n89 = node(w258) -> (w256:dbl)
        n90 = Reciprocal(x=w256) -> (1/x=w253:dbl)
        n91 = node(w257) -> (w255:dbl)
        n92 = Multiply(x=w259, y=w253) -> (x*y=w254:dbl)
        n93 = Add(x=w255, y=w254) -> (x+y=w252:dbl)
        n94 = property on="Measurement" class="WFGraph (strict)"("XScale.Offset"=w255, "XScale.Minimum"=w255, "XScale.Maximum"=w252, "XScale.ScaleFit"=u8 0 ("X Scale.Scale Fit"), "XScale.Multiplier"=w253) -> ()  [unwired: 2 in, 2 out]
        n95 = call-poly <vilib>:"DAQmx Read.vi"("task/channels in"=w275, "error in"=w274) -> ("task out"=w273:refnum<k21>, "data"=w240:dbl[][], "error out"=w272:errorcluster)  [unwired: 11 in]
        n96 = property on="Optical Density Chart" class="WFChart (strict)"() -> ("History Data"=w265:T16)  [unwired: 2 in, 2 out]
        n97 = call "OD Stats Formatter.vi"("OD History"=w265) -> ("Statistics String"=→"Optical Density Signal 1":string, "Statistics String 2"=→"Optical Density Signal 2":string)  [unwired: 9 in, 4 out]
        n98 = call "Numerical Offset and Gain.vi"("Signal 1 Offset"="Signal 1 Offset", "Signal 2 Offset"="Signal 2 Offset", "Signal 1 Gain"="Signal 1 Gain 2", "Signal 2 Gain"="Signal 2 Gain", "Input Data"=w240) -> ("Output Data"=w235:dbl[][])
        n99 = local read "Samples per Channel"() -> (w242:i32)
        n100 = call "2-Ch Optical Density.vi"("Detuning"="Detuning", "Linewidth"="Linewidth", "data"=w235, "Upper Threshold (% of Max)"="Upper Threshold (% of Max)", "Lower Threshold (% of Min)"="Lower Threshold (% of Min)") -> ("Upper Voltage Threshold Reference"=w251:dbl, "Upper Voltage Threshold Signal 1"=w248:dbl, "Upper Voltage Threshold Signal 2"=w244:dbl, "Optical Density 1"=w268:dbl, "Lower Voltage Threshold Reference"=w250:dbl, "Lower Voltage Threshold Signal 1"=w247:dbl, "Lower Voltage Threshold Signal 2"=w245:dbl, "Optical Density 2"=w267:dbl)  [unwired: 3 in]
        n101 = call "Group Reference Toggle.vi"("Samples per Channel"=w242, "Show Reference"="Show Reference", "Show Signal 1"="Show Signal 1", "Show Signal 2"="Show Signal 2", "Upper Voltage Threshold Reference"=w251, "Upper Voltage Threshold Signal 1"=w248, "Lower Voltage Threshold Reference"=w250, "Upper Voltage Threshold Signal 2"=w244, "Lower Voltage Threshold Signal 1"=w247, "Lower Voltage Threshold Signal 2"=w245) -> ("Array"=w241:dbl[][])  [unwired: 2 in, 3 out]
        n102 = Bundle("Optical Density 1"=w268, "Optical Density 2"=w267) -> (→"Optical Density Chart":T5)  [unwired: 1 in]
        n103 = event shown="[1] \"Scan Frequency\": Value Change" {
          selector: _ -> [_ _]
          dyn-events: _ -> [_ _]
          timeout: 0 -> [_ _]
          tunnel: [Raman."Monitor Pulses" ("Raman State") Raman."Scan Frequency" ("Raman State")] -> w271
          event #0 {
            n104 = event-data() -> ()  [unwired: 1 in, 2 out]
          }
          event #1 {
            n105 = event-data() -> ()  [unwired: 1 in, 5 out]
          }
        }
        n106 = Build Array (concatenate)(w235, w241) -> (w234:dbl[][])
        n107 = call "-1 V Offset.vi"("Input Data"=w234) -> ("Output Data"=→"Measurement":dbl[][])
      }
      frame #2 {
        n108 = call "Convert Frequencies.vi"("Resonance Frequency (MHz)"="Resonance Frequency", "Number of Intervals"="Number of Frequency Intervals", "Start Frequency (MHz)"="Start Frequency", "Stop Frequency (MHz)"="Stop Frequency") -> ("Start Frequency (Number)"=w302:dbl, "Frequency Increment (Number)"=w303:dbl, "Number of Intervals (Out)"=w304:u32, "Frequency Interval"=→"Frequency Interval":dbl[unit])
        n109 = for {
          N: w304 -> [_]
          shift-right: [w330] -> w307
          shift-left: w300 -> [w328]
          shift-right: [w331] -> w308
          shift-left: w299 -> [w329]
          tunnel: w303 -> [w325]
          shift-right: [w320] -> _
          shift-left: w302 -> [w312]
          shift-right: [w322] -> w295
          shift-left: w297 -> [w324]
          shift-right: [w321] -> w292
          shift-left: w296 -> [w323]
          tunnel: [w310] -> w285 mode=indexing
          tunnel: [w309] -> w282 mode=indexing
          tunnel: [w315] -> w281 mode=indexing
          n110 = for {
            N: "Number of Measurements" -> [_]
            shift-right: [w344] -> w330
            shift-left: w328 -> [w346]
            shift-right: [w343] -> w331
            shift-left: w329 -> [w345]
            tunnel: [w349] -> w326 mode=indexing
            tunnel: [w348] -> w316 mode=indexing
            i -> [w350]
            stop <- w351 stop-if-true
            w353 = 10.0  # timeout
            # "Acquisition Block"
            # "Send reference into AI0 and Signal into AI1 and AI2"
            n111 = local read "Lower Threshold (% of Min)"() -> (w339:dbl)
            n112 = local read "Upper Threshold (% of Max)"() -> (w340:dbl)
            n113 = local read "Signal 1 Gain 2"() -> (w335:dbl)
            n114 = local read "Signal 1 Offset"() -> (w337:dbl[unit])
            n115 = local read "Signal 2 Offset"() -> (w336:dbl[unit])
            n116 = local read "Linewidth"() -> (w341:dbl[unit])
            n117 = local read "Detuning"() -> (w342:dbl[unit])
            n118 = local read "Signal 2 Gain"() -> (w334:dbl)
            n119 = call-poly <vilib>:"DAQmx Read.vi"("task/channels in"=w346, "timeout"=w353, "error in"=w345) -> ("task out"=w344:refnum<k21>, "data"=w338:dbl[][], "error out"=w343:errorcluster)  [unwired: 10 in]
            n120 = call "Numerical Offset and Gain.vi"("Signal 1 Offset"=w337, "Signal 2 Offset"=w336, "Signal 1 Gain"=w335, "Signal 2 Gain"=w334, "Input Data"=w338) -> ("Output Data"=w333:dbl[][])
            n121 = call "2-Ch Optical Density.vi"("Detuning"=w342, "Linewidth"=w341, "data"=w333, "Upper Threshold (% of Max)"=w340, "Lower Threshold (% of Min)"=w339) -> ("Optical Density 1"=w349:dbl, "Optical Density 2"=w348:dbl)  [unwired: 3 in, 6 out]
            n122 = Unbundle By Name(w343) -> ("status"=w352:bool)
            n123 = call "-1 V Offset.vi"("Input Data"=w333) -> ("Output Data"=w332:dbl[][])
            n124 = local write "Measurement"(w332) -> ()
            n125 = Or(x=w352, y=FALSE) -> (x .or. y?=w351:bool)
            "Acquisition Count" <- w350
          }
          n126 = call <instrlib>:"Config Frequency.vi"("VISA Resource Name"=w324, "Frequency (1000.0)"=w312, "error in (no error)"=w323) -> ("VISA Resource Name Out"=w318:refnum<visa-resource-name>, "error out"=w319:errorcluster)  [unwired: 6 in, 5 out]
          n127 = node(w312) -> (→"Current Frequency":dbl[unit])
          n128 = Add(x=w325, y=w312) -> (x+y=w320:dbl)
          n129 = local read "Resonance Frequency"() -> (w314:dbl[unit])
          n130 = call <instrlib>:"Config Amplitude.vi"("VISA Resource Name"=w318, "Amplitude (-135.00)"=10.0, "error in (no error)"=w319) -> ("VISA Resource Name Out"=w322:refnum<visa-resource-name>, "error out"=w321:errorcluster)  [unwired: 5 in, 6 out]
          n131 = node(w314) -> (w313:dbl)
          n132 = Subtract(x=w312, y=w313) -> (x-y=w309:dbl)
          n133 = call <vilib>:"Std Deviation and Variance.vi"("X"=w326) -> ("mean"=w310:dbl)  [unwired: 1 in, 2 out]
          n134 = call <vilib>:"Std Deviation and Variance.vi"("X"=w316) -> ("mean"=w315:dbl)  [unwired: 1 in, 2 out]
        }
        n135 = local read "Resonance Frequency"() -> (w283:dbl[unit])
        n136 = Bundle(w282, w281) -> (w287:cluster{dbl[], dbl[]})  [unwired: 1 in]
        n137 = Bundle(w282, w285) -> (w288:cluster{dbl[], dbl[]})  [unwired: 1 in]
        n138 = Build Array(w282, w285, w281) -> (w284:dbl[][])
        n139 = Build Array(w288, w287) -> (→"Raman Measure - Frequency Scan":cluster{dbl[], dbl[]}[])
        n140 = local write "Current Frequency"(w283) -> ()
        n141 = node(w283) -> (w291:dbl)
        n142 = call <instrlib>:"Config Frequency.vi"("VISA Resource Name"=w295, "Frequency (1000.0)"=w291, "error in (no error)"=w292) -> ("VISA Resource Name Out"=w294:refnum<visa-resource-name>, "error out"=w293:errorcluster)  [unwired: 6 in, 5 out]
      }
      frame #3 {
        n143 = local read "Raman Measurement File Root"() -> (w356:path)
        n144 = call "Add Timestamp to File and Directory.vi"("File Path"=w356) -> ("appended path"=w355:path)  [unwired: 1 in]
        n145 = call-poly <vilib>:"Write To Spreadsheet File.vi"("transpose? (no:F)"=TRUE, "format (%.3f)"="%.9f", "2D data"=w362, "file path (dialog if empty)"=w355) -> ("new file path (Not A Path if cancelled)"=→"Raman Measurement File":path)  [unwired: 4 in]
      }
      frame #4 {
        # "Do nothing, remain in standby state"
      }
      frame #5 {
        w370 = T13 3 items=["no dialog", "OK message", "continue or stop message", "OK message + warnings", "continue/stop + warnings"] ("type of dialog (OK msg:1)")
        # "Stop and clear acquisition task, and transition \ninto a standby state"
        n146 = call <vilib>:"DAQmx Clear Task.vi"("task in"=w384, "error in"=w383) -> ("error out"=w385:errorcluster)  [unwired: 13 in]
        n147 = call <vilib>:"Simple Error Handler.vi"("type of dialog (OK msg:1)"=w370, "error in (no error)"=w385) -> ("error out"=w382:errorcluster)  [unwired: 3 in, 4 out]
        n148 = call <instrlib>:"RF On_OFF.vi"("VISA Resource Name"=w372, "error in (no error)"=w371) -> ("VISA Resource Name Out"=w377:refnum<visa-resource-name>, "error out"=w378:errorcluster)  [unwired: 1 in, 11 out]
        n149 = call <instrlib>:"Error Query.vi"("VISA Resource Name"=w377, "error in (no error)"=w378) -> ("VISA Resource Name Out"=w376:refnum<visa-resource-name>, "error out"=w379:errorcluster)  [unwired: 12 out]
        n150 = call <instrlib>:"Error Message.vi"("VISA Resource Name"=w376, "error in (no error)"=w379) -> ("VISA Resource Name Out"=w375:refnum<visa-resource-name>, "error out"=w380:errorcluster)  [unwired: 1 in, 11 out]
        n151 = call <instrlib>:"Close.vi"("VISA Resource Name"=w375, "error in (no error)"=w380) -> ()  [unwired: 14 out]
      }
    }
  }
  n152 = disable-structure shown="Disabled" {
    disable-tunnel: w1 -> [w387 _]
    frame #0 {
      n153 = while {
        tunnel: w387 -> [w443]
        stop <- w444 stop-if-true
        w423 = 1000.0 ("x")
        n154 = local read "Memory Repetition Period"() -> (w422:dbl[unit])
        n155 = local read "Reference Pulse"() -> (w441:dbl[])
        n156 = Dequeue Element(queue=w443, timeout in ms (-1)=1000) -> (element=w403:dbl[])  [unwired: 1 in, 3 out]
        n157 = Build Array(w403, w441) -> (→"Acquisition Sequence":dbl[][])
        n158 = node(w422) -> (w437:dbl)
        n159 = property on="Risetime Chart" class="WFChart (strict)"("XScale.Multiplier"=w437) -> ("History Data"=w436:cluster{dbl}[])  [unwired: 2 in, 2 out]
        n160 = property on="Falltime Chart" class="WFChart (strict)"("XScale.Multiplier"=w437) -> ("History Data"=w431:cluster{dbl}[])  [unwired: 2 in, 2 out]
        n161 = property on="Width Chart" class="WFChart (strict)"("XScale.Multiplier"=w437) -> ("History Data"=w426:cluster{dbl}[])  [unwired: 2 in, 2 out]
        n162 = property on="Delay Chart" class="WFChart (strict)"("XScale.Multiplier"=w437) -> ("History Data"=w425:cluster{dbl}[])  [unwired: 2 in, 2 out]
        n163 = property on="Amplitude Chart" class="WFChart (strict)"("XScale.Multiplier"=w437) -> ("History Data"=w424:cluster{dbl}[])  [unwired: 2 in, 2 out]
        n164 = local read "Acquisitions Remaining"() -> (w440:i32)
        n165 = call "Stats Formatter.vi"("Unit String"=" ns" ("string"), "History Data"=w436, "factor"=w423) -> ("Statistics String"=→"Risetime":string)  [unwired: 2 out]
        n166 = call "Stats Formatter.vi"("Unit String"=" ns" ("string"), "History Data"=w431, "factor"=w423) -> ("Statistics String"=→"Falltime":string)  [unwired: 2 out]
        n167 = call "Stats Formatter.vi"("History Data"=w426) -> ("Statistics String"=→"Pulse Width":string)  [unwired: 2 in, 2 out]
        n168 = call "Stats Formatter.vi"("History Data"=w425) -> ("Statistics String"=→"Delay":string, "Mean"=w402:dbl)  [unwired: 2 in, 1 out]
        n169 = call "Stats Formatter.vi"("Unit String"=" V" ("string"), "History Data"=w424) -> ("Statistics String"=→"Amplitude":string)  [unwired: 1 in, 2 out]
        n170 = Greater Than 0?(x=w440) -> (x > 0?=w439:bool)
        n171 = case shown="True" w439 {
          tunnel: [_ TRUE ("Blinking")] -> w438
          tunnel: w440 -> [_ w452]
          tunnel: w403 -> [_ w448]
          frame #0 {
            n172 = local write "Writing Phase to File"(FALSE ("Save to File")) -> ()
          }
          frame #1 {
            n173 = local read "Quadrature Pulses File"() -> (w451:path)
            n174 = Decrement(x=w452) -> (x-1=w454:i32)
            n175 = local write "Acquisitions Remaining"(w454) -> ()
            n176 = call-poly <vilib>:"Write To Spreadsheet File.vi"("format (%.3f)"="%.9f", "append to file? (new file:F)"=TRUE, "1D data"=w448, "file path (dialog if empty)"=w451) -> ()  [unwired: 2 in, 3 out]
          }
        }
        n177 = local read "Actual Sample Rate"() -> (w419:dbl[unit])
        n178 = Reciprocal(x=w419) -> (1/x=w405:dbl[unit])
        "Interval Between Samples" <- w405
        n179 = property on="Acquire Data" class="Bool (strict)"("Blinking"=w438) -> ()  [unwired: 2 in, 2 out]
        n180 = call <vilib>:"Pulse Parameters.vi"("X"=w403) -> ("risetime"=w415:dbl, "amplitude"=w420:dbl, "delay"=w418:dbl, "duration"=w417:dbl, "falltime"=w416:dbl)  [unwired: 10 out]
        n181 = node(w405) -> (w404:dbl)
        n182 = local read "Number of Samples per Pulse"() -> (w401:i32)
        n183 = property on="Acquisition Sequence" class="WFGraph (strict)"("XScale.Multiplier"=w404) -> ()  [unwired: 2 in, 2 out]
        n184 = Multiply(x=w404, y=w417) -> (x*y=w407:dbl)
        n185 = Multiply(x=w404, y=w418) -> (x*y=w406:dbl)
        n186 = Multiply(x=w404, y=w416) -> (x*y=w408:dbl)
        n187 = Multiply(x=w404, y=w415) -> (x*y=w414:dbl)
        n188 = Less Than 0?(x=w420) -> (x < 0?=w421:bool)
        n189 = Bundle(w414) -> (→"Risetime Chart":cluster{dbl})  [unwired: 1 in]
        n190 = Bundle(w408) -> (→"Falltime Chart":cluster{dbl})  [unwired: 1 in]
        n191 = Bundle(w407) -> (→"Width Chart":cluster{dbl})  [unwired: 1 in]
        n192 = Bundle(w406) -> (→"Delay Chart":cluster{dbl})  [unwired: 1 in]
        n193 = Bundle("amplitude"=w420) -> (→"Amplitude Chart":cluster{"amplitude":dbl})  [unwired: 1 in]
        n194 = case shown="True" w421 {
          tunnel: w402 -> [_ w446]
          frame #0 {
          }
          frame #1 {
            # "Time needed to add to EIT \nsignal delay since pulse doesn't start \nright when we recieve trigger"
            n195 = node(w446) -> (→"Global EIT Delay":dbl[unit])
          }
        }
        n196 = local read "Actual Sample Rate"() -> (w400:dbl[unit])
        n197 = local read "Memory Repetition Period"() -> (w389:dbl[unit])
        n198 = local read "Acquisition Delay"() -> (w393:dbl[unit])
        n199 = call "Timing Helper.vi"("Repetition Period"=w389, "Number of points per run"=w401, "Number of runs"="Number of Pulses to Record", "Sample rate"=w400) -> ("Total Experiment Time"=→"Total Experiment Time":dbl[unit], "Total Number of Datapoints"=→"Total Number of Datapoints":i64, "Total Acquired Time"=→"Total Acquired Time":dbl[unit], "Acquisition Time per Run"=w398:dbl[unit])
        n200 = Add(x=w393, y=w398) -> (x+y=w394:dbl[unit])
        n201 = node(w393) -> (w390:dbl)
        n202 = node(w394) -> (w391:dbl)
        n203 = local read "Master Stop"() -> (w444:bool)
        n204 = property on="Acquisition Sequence" class="WFGraph (strict)"("XScale.Offset"=w390, "XScale.Minimum"=w390, "XScale.ScaleFit"=u8 0 ("X Scale.Scale Fit"), "XScale.Maximum"=w391) -> ()  [unwired: 2 in, 2 out]
      }
    }
    frame #1 {
    }
  }
  n205 = Obtain Queue(name (unnamed)="Phase", element data type=dbl[][] [] ("data")) -> (queue out=w26:refnum<queue>)  [unwired: 3 in, 2 out]
  n206 = disable-structure shown="Disabled" {
    disable-tunnel: w60 -> [w460 _]
    disable-tunnel: w59 -> [w459 _]
    disable-tunnel: w58 -> [w458 _]
    disable-tunnel: [w457 _] -> w33
    disable-tunnel: w1 -> [w455 _]
    frame #0 {
      n207 = while {
        shift-right: [w470] -> _
        shift-left: w458 -> [w468]
        shift-right: [w477] -> w462
        shift-left: w460 -> [w475]
        shift-right: [w476] -> w456
        shift-left: w459 -> [w474]
        shift-right: [w473] -> _
        shift-left: _ -> [w472]
        shift-right: [w467] -> _
        shift-left: FALSE -> [w466]
        tunnel: w455 -> [w464]
        stop <- w471 stop-if-true
        # "Pulse  Acquisition Loop"
        n208 = local read "Master Stop"() -> (w465:bool)
        n209 = case shown="False" w465 {
          tunnel: [w479 5122-States."Exit" ("Enum")] -> w469
          tunnel: w468 -> [w482 _]
          frame #0 {
            n210 = case shown="\"Initialize Card\", Default" w482 {
              selector: w482 -> [w483 w484 w485 w486 w487 _]
              tunnel: [w483 w484 w485 w486 w487 5122-States."Initialize Card" ("Enum")] -> w481
              frame #0 {
              }
              frame #1 {
              }
              frame #2 {
              }
              frame #3 {
              }
              frame #4 {
              }
              frame #5 {
              }
            }
            n211 = Select(t=w481, s="Acquire Data", f=5122-States."Standby" ("Enum")) -> (s? t:f=w479:T15)
          }
          frame #1 {
          }
        }
        n212 = case shown="\"Initialize Card\", Default" w469 {
          selector: w469 -> [_ _ _ _ w599]
          tunnel: [w506 w544 w558 w597 w600] -> w477
          tunnel: [w504 w545 w552 w596 w601] -> w476
          tunnel: w475 -> [w509 w547 w557 w597 w600]
          tunnel: w474 -> [w508 w546 w556 w596 w601]
          tunnel: [5122-States."Continuous Mode" ("Enum") 5122-States."Fetch" ("Enum") w550 _ w599] -> w470
          tunnel: [_ _ _ TRUE ("Acquire Data") _] -> w471
          tunnel: [_ _ w553 _ _] -> w473
          tunnel: w472 -> [_ _ _ _ _]
          tunnel: [TRUE w542 _ _ _] -> w467
          tunnel: w466 -> [_ w542 w549 _ _]
          tunnel: w464 -> [_ _ w548 _ _]
          frame #0 {
            w491 = u8 0 ("Disabled")
            w518 = 0 items=["Positive", "Negative"] ("Trigger slope 6")
            w525 = TRUE  # Enforce realtime
            w515 = 1.0  # Probe attenuation
            w521 = u32 0 items=["1 mega ohm", "75 ohms", "50 ohms"]  # Input impedance
            # "Desired Number of Samples"
            n213 = property on="Capture" class="Bool"("Disabled"=w491) -> ()  [unwired: 2 in, 2 out]
            n214 = property on="Total Acquired Time" class="DigNum (strict)"("Disabled"=w491) -> ()  [unwired: 2 in, 2 out]
            n215 = property on="Acquisition Sequence" class="WFGraph (strict)"("Disabled"=w491) -> ()  [unwired: 2 in, 2 out]
            n216 = property on="Total Experiment Time" class="DigNum (strict)"("Disabled"=w491) -> ()  [unwired: 2 in, 2 out]
            n217 = property on="Acquisitions Remaining" class="DigNum (strict)"("Disabled"=w491) -> ()  [unwired: 2 in, 2 out]
            n218 = property on="Number of Pulses to Record" class="DigNum (strict)"("Disabled"=w491) -> ()  [unwired: 2 in, 2 out]
            n219 = property on="Acquisition Time per Pulse" class="DigNum (strict)"("Disabled"=w491) -> ()  [unwired: 2 in, 2 out]
            n220 = property on="Channel" class="Ring (strict)"("Disabled"=w491) -> ()  [unwired: 2 in, 2 out]
            n221 = property on="Vertical coupling" class="Ring (strict)"("Disabled"=w491) -> ()  [unwired: 2 in, 2 out]
            n222 = property on="Vertical range (0 to 10V)" class="DigNum (strict)"("Disabled"=w491) -> ()  [unwired: 2 in, 2 out]
            n223 = property on="Desired Sample Rate" class="DigNum (strict)"("Disabled"=w491) -> ()  [unwired: 2 in, 2 out]
            n224 = property on="Acquisition Delay" class="DigNum (strict)"("Disabled"=w491) -> ()  [unwired: 2 in, 2 out]
            n225 = property on="Get Reference Parameters" class="Bool"("Disabled"=w491) -> ()  [unwired: 2 in, 2 out]
            n226 = disable-structure shown="Enabled" {
              frame #0 {
                w527 = 0
                n227 = property on="Falltime Chart" class="WFChart (strict)"("XScale.Minimum"=w527) -> ()  [unwired: 2 in, 2 out]
                n228 = property on="Width Chart" class="WFChart (strict)"("XScale.Minimum"=w527) -> ()  [unwired: 2 in, 2 out]
                n229 = property on="Risetime Chart" class="WFChart (strict)"("XScale.Minimum"=w527) -> ()  [unwired: 2 in, 2 out]
                n230 = property on="Amplitude Chart" class="WFChart (strict)"("XScale.RngStart"=w527) -> ()  [unwired: 2 in, 2 out]
                n231 = property on="Delay Chart" class="WFChart (strict)"("XScale.RngStart"=w527) -> ()  [unwired: 2 in, 2 out]
              }
              frame #1 {
              }
            }
            n232 = node("Vertical range (0 to 10V)") -> (w497:dbl)
            n233 = Number To Decimal String(number="Channel") -> (decimal integer string=w510:string)  [unwired: 1 out]
            "Channel String" <- w510
            n234 = property on="Acquire Phase" class="Bool (strict)"("Val(Sgnl)"=TRUE ("Value (Signaling)")) -> ()  [unwired: 2 in, 2 out]
            n235 = node("Desired Sample Rate") -> (w502:dbl)
            n236 = local write "Acquisitions Remaining"(0 ("Acquisitions Remaining")) -> ()
            n237 = Multiply(x="Desired Sample Rate", y="Acquisition Time per Pulse") -> (x*y=w498:dbl)
            n238 = node(dbl[unit] 0.5 ("Trigger level")) -> (w512:dbl)
            n239 = case shown="1" "Vertical coupling" {
              tunnel: w497 -> [w532 w537 w540]
              tunnel: [0 0.0 w538] -> w494
              frame #0 {
                n240 = Divide(x=w532, y=2.0) -> (x/y=w530:dbl)
                n241 = Negate(x=w530) -> (-x=w529:dbl)
                n242 = property on="Acquisition Sequence" class="WFGraph (strict)"("YScale.Maximum"=w530, "YScale.Minimum"=w529) -> ()  [unwired: 2 in, 2 out]
              }
              frame #1 {
                n243 = Divide(x=w537, y=2.0) -> (x/y=w535:dbl)
                n244 = Negate(x=w535) -> (-x=w534:dbl)
                n245 = property on="Acquisition Sequence" class="WFGraph (strict)"("YScale.Maximum"=w535, "YScale.Minimum"=w534) -> ()  [unwired: 2 in, 2 out]
              }
              frame #2 {
                n246 = Divide(x=w540, y=2.0) -> (x/y=w538:dbl)
                n247 = property on="Acquisition Sequence" class="WFGraph (strict)"("YScale.Maximum"=w540, "YScale.Minimum"=0.0 ("Y Scale.Range:Minimum")) -> ()  [unwired: 2 in, 2 out]
              }
            }
            n248 = call <instrlib>:"niScope Configure Vertical.vi"("instrument handle"=w509, "probe attenuation"=w515, "vertical coupling"="Vertical coupling", "channels"=w510, "vertical range"=w497, "vertical offset"=w494, "error in"=w508) -> ("instrument handle out"=w524:refnum<k15>, "error out"=w523:errorcluster)  [unwired: 1 in, 6 out]
            n249 = call <instrlib>:"niScope Configure Chan Characteristics.vi"("instrument handle"=w524, "channels"=w510, "input impedance"=w521, "error in"=w523) -> ("instrument handle out"=w516:refnum<k15>, "error out"=w522:errorcluster)  [unwired: 1 in, 9 out]
            n250 = call <instrlib>:"niScope Configure Horizontal Timing.vi"("instrument handle"=w516, "enforce realtime"=w525, "min sample rate"=w502, "reference position"=0.0, "error in"=w522, "min record length"=w498) -> ("instrument handle out"=w519:refnum<k15>, "error out"=w520:errorcluster)  [unwired: 1 in, 7 out]
            n251 = node("Acquisition Delay") -> (w503:dbl)
            n252 = call-poly <instrlib>:"niScope Configure Trigger (poly).vi"("instrument handle"=w519, "trigger slope"=w518, "trigger source"="VAL_EXTERNAL" ("Trigger source"), "trigger level"=w512, "error in"=w520, "trigger delay"=w503) -> ("instrument handle out"=w507:refnum<k15>, "error out"=w505:errorcluster)  [unwired: 2 in, 6 out]
            n253 = call <instrlib>:"niScope Commit.vi"("instrument handle"=w507, "error in"=w505) -> ("instrument handle out"=w506:refnum<k15>, "error out"=w504:errorcluster)  [unwired: 12 out]
          }
          frame #1 {
            n254 = call <instrlib>:"niScope Initiate Acquisition.vi"("instrument handle"=w547, "error in"=w546) -> ("instrument handle out"=w544:refnum<k15>, "error out"=w545:errorcluster)  [unwired: 12 out]
          }
          frame #2 {
            # "clear file"
            n255 = call <instrlib>:"niScope Acquisition Status.vi"("instrument handle"=w557, "error in"=w556) -> ("instrument handle out"=w555:refnum<k15>, "acquisition status"=w551:i32, "error out"=w554:errorcluster)  [unwired: 11 out]
            n256 = case shown="1" w551 {
              tunnel: [w561 w566] -> w558
              tunnel: w555 -> [w561 w581]
              tunnel: w554 -> [w560 w579]
              tunnel: [_ w563] -> w553
              tunnel: [5122-States."Fetch" ("Enum") w576] -> w550
              tunnel: [w560 w567] -> w552
              tunnel: w549 -> [_ _]
              tunnel: w548 -> [_ w562]
              frame #0 {
              }
              frame #1 {
                n257 = call <instrlib>:"niScope Actual Record Length.vi"("instrument handle"=w581, "error in"=w579) -> ("instrument handle out"=w580:refnum<k15>, "actual record length"=→"Number of Samples per Pulse":i32, "error out"=w571:errorcluster)  [unwired: 11 out]
                n258 = call <instrlib>:"niScope Sample Rate.vi"("instrument handle"=w580, "error in"=w571) -> ("instrument handle out"=w572:refnum<k15>, "actual sample rate"=w569:dbl, "error out"=w570:errorcluster)  [unwired: 11 out]
                n259 = node(w569) -> (→"Actual Sample Rate":dbl[unit])
                n260 = local read "Channel String"() -> (w574:string)
                n261 = call-poly <instrlib>:"niScope Fetch (poly).vi"("timeout"=0.0, "error in"=w570, "channels"=w574, "instrument handle"=w572) -> ("error out"=w567:errorcluster, "wfm"=w563:dbl[], "instrument handle out"=w566:refnum<k15>)  [unwired: 1 in, 4 out]
                n262 = event shown="[1] \"Capture\": Value Change" {
                  selector: _ -> [_ _ _ _]
                  dyn-events: _ -> [_ _ _ _]
                  timeout: 0 -> [_ _ _ _]
                  tunnel: [5122-States."Continuous Mode" ("Enum") 5122-States."Continuous Mode" ("Enum") 5122-States."Initialize Card" ("Enum") 5122-States."Continuous Mode" ("Enum")] -> w564
                  tunnel: w563 -> [_ _ _ w592]
                  event #0 {
                    n263 = event-data() -> ()  [unwired: 3 out]
                  }
                  event #1 {
                    w585 = T9."replace or create" ("operation (0:open)")
                    n264 = event-data() -> ()  [unwired: 2 out]
                    n265 = local read "Raw Phase, Trigger, Extracted Phase Data"() -> (w584:path)
                    n266 = local read "Phase-Frequency Pairs"() -> (w583:path)
                    n267 = local read "Quadrature Pulses File"() -> (w586:path)
                    n268 = Open/Create/Replace File(file path (use dialog)=w586, operation (0:open)=w585) -> ()  [unwired: 4 in, 3 out]
                    n269 = Open/Create/Replace File(file path (use dialog)=w583, operation (0:open)=w585) -> ()  [unwired: 4 in, 3 out]
                    n270 = Open/Create/Replace File(file path (use dialog)=w584, operation (0:open)=w585) -> ()  [unwired: 4 in, 3 out]
                    n271 = local read "Number of Pulses to Record"() -> (→"Acquisitions Remaining":i32)
                    n272 = local write "Writing Phase to File"(TRUE ("Write Phase to File")) -> ()
                  }
                  event #2 {
                    n273 = event-data() -> ()  [unwired: 3 out]
                  }
                  event #3 {
                    n274 = event-data() -> ()  [unwired: 5 out]
                    n275 = local read "Reference Pulse File"() -> (w591:path)
                    n276 = call-poly <vilib>:"Write To Spreadsheet File.vi"("format (%.3f)"="%.9f", "1D data"=w592, "file path (dialog if empty)"=w591) -> ()  [unwired: 3 in, 3 out]
                    "Reference Pulse" <- w592
                  }
                }
                n277 = Enqueue Element(queue=w562, element=w563) -> ()  [unwired: 2 in, 3 out]
                n278 = Unbundle By Name(w567) -> ("status"=w577:bool)
                n279 = Select(t=5122-States."Exit" ("Enum"), s=w577, f=w564) -> (s? t:f=w576:T15)
              }
            }
          }
          frame #3 {
          }
          frame #4 {
            w598 = u8 2 ("Disabled")
            n280 = property on="Acquisition Time per Pulse" class="DigNum (strict)"("Disabled"=w598) -> ()  [unwired: 2 in, 2 out]
            n281 = property on="Capture" class="Bool"("Disabled"=w598) -> ()  [unwired: 2 in, 2 out]
            n282 = property on="Total Acquired Time" class="DigNum (strict)"("Disabled"=w598) -> ()  [unwired: 2 in, 2 out]
            n283 = property on="Acquisition Sequence" class="WFGraph (strict)"("Disabled"=w598) -> ()  [unwired: 2 in, 2 out]
            n284 = property on="Total Experiment Time" class="DigNum (strict)"("Disabled"=w598) -> ()  [unwired: 2 in, 2 out]
            n285 = property on="Number of Pulses to Record" class="DigNum (strict)"("Disabled"=w598) -> ()  [unwired: 2 in, 2 out]
            n286 = property on="Channel" class="Ring (strict)"("Disabled"=w598) -> ()  [unwired: 2 in, 2 out]
            n287 = property on="Vertical coupling" class="Ring (strict)"("Disabled"=w598) -> ()  [unwired: 2 in, 2 out]
            n288 = property on="Vertical range (0 to 10V)" class="DigNum (strict)"("Disabled"=w598) -> ()  [unwired: 2 in, 2 out]
            n289 = property on="Desired Sample Rate" class="DigNum (strict)"("Disabled"=w598) -> ()  [unwired: 2 in, 2 out]
            n290 = property on="Acquisition Delay" class="DigNum (strict)"("Disabled"=w598) -> ()  [unwired: 2 in, 2 out]
            n291 = property on="Acquisitions Remaining" class="DigNum (strict)"("Disabled"=w598) -> ()  [unwired: 2 in, 2 out]
            n292 = property on="Get Reference Parameters" class="Bool"("Disabled"=w598) -> ()  [unwired: 2 in, 2 out]
          }
        }
      }
      n293 = call <instrlib>:"niScope Close.vi"("instrument handle"=w462, "error in"=w456) -> ("error out"=w463:errorcluster)  [unwired: 13 out]
      n294 = call <vilib>:"Simple Error Handler.vi"("error in (no error)"=w463) -> ("error out"=w457:errorcluster)  [unwired: 1 in, 7 out]
    }
    frame #1 {
    }
  }
  n295 = while {
    tunnel: [w605] -> w20
    tunnel: w26 -> [w603]
    stop <- w604 stop-if-true
    # "Phase Writing Loop"
    n296 = local read "Acquire Phase"() -> (w602:bool)
    n297 = local read "Master Stop"() -> (w604:bool)
    n298 = case shown="True" w602 {
      tunnel: [w606 w610] -> w605
      tunnel: w603 -> [w606 w611]
      frame #0 {
      }
      frame #1 {
        # "Only proceed if There are data point to plot/record"
        n299 = Dequeue Element(queue=w611, timeout in ms (-1)=1000) -> (queue out=w610:refnum<queue>, element=w609:dbl[][], timed out?=w608:bool)  [unwired: 1 in, 1 out]
        n300 = case shown="False" w608 {
          tunnel: w610 -> [_ _]
          tunnel: w609 -> [w613 _]
          frame #0 {
            n301 = local read "Phase Acquisition Sampling Freq"() -> (w615:dbl)
            n302 = local read "samples per channel"() -> (w617:i32)
            n303 = Reciprocal(x=w615) -> (1/x=w614:dbl)
            n304 = Bundle("Phase Acquisition Sampling Freq"=w615, "samples per channel"=w617) -> (w616:T17)  [unwired: 1 in]
            n305 = call "Create RawPhase, TTL, Extracted Phase from Raw Phase Data.vi"("sampling info"=w616, "sampling freq: fs"=w615, "Raw Input Data"=w613, "order"="Filter Order", "dt"=w614, "low cutoff freq: fl"="Low Pass Filter Cutoff Freq: Hz") -> ("detected frequency"=→"detected frequency":dbl, "Output Data"=w622:dbl[][], "Phase Frequency Pairs"=w612:dbl[][], "Normalized Envelope"=→"Normalized Envelope":waveform(dbl))  [unwired: 2 in, 4 out]
            "Phase Monitor" <- w622
            "Phase Frequency Pairs" <- w612
            n306 = local read "Writing Phase to File"() -> (w623:bool)
            n307 = case shown="True" w623 {
              tunnel: w622 -> [_ _]
              tunnel: w612 -> [_ w624]
              frame #0 {
              }
              frame #1 {
                w627 = TRUE ("transpose? (no:F)")
                w628 = "%.9f" ("format (%.3f)")
                w629 = TRUE ("transpose? (no:F)")
                # "Send in Memory Sequence Trig for now.  (Who trigs 5122) \nIts not accurate, but its not important.  \nWe care about relative phase, not absolute\nChange later by sending a trig right before memmory pulse is created"
                # "File Format: Raw Phase, Sqz Measurement Trig (TTL), and Arches Data"
                # "Extracted Phases corresponding to\n Quadrature  Measurements"
                n308 = local read "Phase-Frequency Pairs"() -> (w625:path)
                n309 = local read "Raw Phase, Trigger, Extracted Phase Data"() -> (w626:path)
                n310 = call-poly <vilib>:"Write To Spreadsheet File.vi"("transpose? (no:F)"=w629, "format (%.3f)"=w628, "append to file? (new file:F)"=w629, "file path (dialog if empty)"=w626) -> ()  [unwired: 4 in, 1 out]
                n311 = call-poly <vilib>:"Write To Spreadsheet File.vi"("transpose? (no:F)"=w627, "format (%.3f)"=w628, "append to file? (new file:F)"=w627, "2D data"=w624, "file path (dialog if empty)"=w625) -> ()  [unwired: 3 in, 1 out]
              }
            }
          }
          frame #1 {
          }
        }
      }
    }
  }
  n312 = xnode "Open FPGA VI Reference"("resource name"="FPGA Target") -> ("FPGA VI Reference Out"=w44:refnum<k20>, "error out"=w42:errorcluster)  [unwired: 1 in]
  n313 = while {
    shift-right: [w631] -> _
    shift-left: States."Initialize" ("Enum") -> [w637]
    tunnel: w44 -> [w636]
    tunnel: w42 -> [w635]
    tunnel: [w634] -> w47
    tunnel: [w633] -> w46
    stop <- w630 stop-if-true
    # "FPGA Timing Loop"
    n314 = case shown="\"Send Data\"" w637 {
      selector: w637 -> [_ _ _ w1066 _ _]
      tunnel: w636 -> [w642 w722 w1058 w1070 w1326 w2805]
      tunnel: w635 -> [w639 w721 w1057 w1064 w1325 w2804]
      tunnel: [w640 w715 w1058 w1069 w1327 w2805] -> w634
      tunnel: [w638 w714 w1057 w1068 w1322 w2804] -> w633
      tunnel: [_ _ _ w1062 _ _] -> w630
      tunnel: [States."Send Data" ("Enum") States."Check for Activity" ("Enum") w1052 w1066 w1319 States."Check for Activity" ("Enum")] -> w631
      frame #0 {
        n315 = disable-structure shown="Enabled" {
          disable-tunnel: w642 -> [w648 w683]
          disable-tunnel: [w647 w683] -> w640
          disable-tunnel: w639 -> [w645 w682]
          disable-tunnel: [w644 w682] -> w638
          frame #0 {
            n316 = xnode "Invoke Method"("FPGA VI Reference In"=w648, "error in"=w645, "Depth"=u32 400000) -> ("FPGA VI Reference Out"=w647:refnum<k20>, "error out"=w644:errorcluster)
          }
          frame #1 {
          }
        }
        n317 = property on="Active" class="Bool (strict)"("Blinking"=TRUE) -> ()  [unwired: 2 in, 2 out]
      }
      frame #1 {
        n318 = xnode "Read/Write Control"("FPGA VI Reference In"=w722, "error in"=w721) -> ("FPGA VI Reference Out"=w715:refnum<k20>, "error out"=w714:errorcluster, "Last Global Period"=w719:u64, "Last Memory Period"=w713:u64, "Last DLCZ Period"=w711:u64, "Global Time"=w709:u64, "Memory Timer"=w707:u64, "Memory Mode"=→"Memory Mode 2":T4, "Current State"=→"Current State":T8, "Raman/OD Acquisition Delay"=w705:u64, "SPME Start"=w703:u64, "SPME Control - stop"=w701:u64, "SPME Control - start"=w699:u64, "Num of SPME Pulses per Mem Seq"=→"Read Num of SPME Pulses per Mem Seq":u64, "SPME Signal start"=w696:u64, "SPME Period"=w694:u64, "SPME Signal stop"=w692:u64, "Last SPME Interval between Resets"=w689:u64, "SPME Count"=→"SPME Count":u64, "Last N1"=→"N1":u64, "Current N1"=→"N2":u64, "Number of Trials"=→"Number of Trials":u64)
        n319 = call "Convert Ticks to Time.vi"("Ticks"=w719, "Ticks 2"=w713, "Ticks 3"=w711, "Ticks 4"=w709, "Ticks 5"=w707, "Ticks 6"=w705) -> ("Time"=→"Measured Acquisition Rate":dbl[unit], "Time  2"=→"Measured Memory Sequence Duration":dbl[unit], "Time  3"=→"Last DLCZ Period":dbl[unit], "Time  4"=→"Global Time":dbl[unit], "Time  5"=→"Memory Timer":dbl[unit], "Time  6"=→"Raman/OD Aquisition Delay":dbl[unit])  [unwired: 14 in, 2 out]
        n320 = call "Convert Ticks to Time.vi"("Ticks"=w703, "Ticks 2"=w701, "Ticks 3"=w699, "Ticks 4"=w696, "Ticks 5"=w694, "Ticks 6"=w692, "Ticks 7"=w689) -> ("Time"=→"Read SPME Start":dbl[unit], "Time  2"=→"Read SPME Control Stop":dbl[unit], "Time  3"=→"Read SPME Control Start":dbl[unit], "Time  4"=→"Read SPME Signal Start":dbl[unit], "Time  5"=→"Read SPME Period":dbl[unit], "Time  6"=→"Read SPME Signal Stop":dbl[unit], "Time  7"=→"Last SPME Interval Between Resets":dbl[unit], "Time  8"=→"Memory Acquisition Trigger Delay":dbl[unit])  [unwired: 13 in]
      }
      frame #2 {
        n321 = event shown="[1] \"Control Duration (DIO5/1) \", \"Pump (DIO19) \", \"Repump (DIO18)\", \"Coherent Signal Delay (DIO6)\", \"Coherent Signal Duration (DIO6)\", \"Output  Trigger Sign (DIO13)\", \"DLCZ Pulse Duration\", \" DLCZ Period\", \"Opt Density Duration (DIO7)\", \"Opt Density Delay (DIO7)\", \"Trapping (DIO17)\", \"Memory Mode\", \"Control Delay(DIO5/1)\", \" DLCZ Start\", \" DLCZ Stop\", \"A\", \"B\", \"Global Delay\", \"Raman Signal Duration (DIO6)\", \"Raman Signal Delay (DIO6)\", \"Raman Control Delay(DIO5)\", \"Ramand Control Duration (DIO5) \", \"SQZ AOM Signal Duration (DIO6)\", \"SQZ AOM Signal Delay (DIO6)\", \" OD Acquisition Delay \", \"SPME Control Delay(DIO5/1)\", \"SPME Control Duration (DIO5/1)\", \"SPME Signal Duration (DIO5/1)\", \"SPME Signal Delay(DIO5/1)\", \"Num of SPME Pulses per Mem Seq\", \"SPME Period\", \"SPME Start\", \"SPME Leakage Gate Delay\", \"SPME Leakage Gate Duration\", \"SPME Signal Gate Delay\", \"SPME Signal Gate Duration\", \"Desired Number of Trials\", \"Memory\", \"WA Control 1 (DIO4)\", \"WA Control 1 (DIO4)\", \"WA Control 2 (DIO4)\", \"WA Control 2 (DIO4)\", \"WA Pump (DIO2)\", \"WA Pump (DIO2)\", \"WA Repump (DIO3)\", \"WA Repump (DIO3)\", \"WA Signal (DIO5)\", \"WA Signal (DIO5)\", \"WA Control Switch 1 (DIO6) \", \"WA Control Switch 1(DIO6)\", \"WA ControlS 2 (DIO6) \", \"WA ControlS 2 (DIO6) \", \"WA Control Sign\", \"WA Pump Sign\", \"WA Repump Sign\", \" WA Signal Sign\", \"WA Output  Trigger  Sign (DIO1)\", \"WA ControlS Sign\", \"WA Repetition Period\", \"Coherent Signal Sign\", \"SQZ AOM Control Sign \", \"Raman Control Sign \", \"Raman Signal Sign\", \"DLCZ Sign\", \"SPME Control Sign\", \"SPME Signal Sign\", \"SPME Gate1 Sign\", \"SPME Gate2 Sign\", \"OD Sign\", \"SQZ AOM Signal Sign\", \"Coherent Control Sign\", \"WA Signal Switch (DIO7)\", \"WA Signal Switch (DIO7)\", \" WA Signal Switch Sign\", \"WA Signal Switch 2 (DIO7)\", \"WA Signal Switch 2  (DIO7)\", \"WA Extra (DIO0)\", \"WA Extra  (DIO0)\", \" WA Extra Sign\", \"WA Extra 2 (DIO0) \", \"WA Extra 2 (DIO0)\", \"WA Extra 3 (DIO0)\", \"WA Extra 3 (DIO0)\", \"WA Extra 4 (DIO0) \", \"WA Extra 4 (DIO0)\", \"Memory Acquisition Trigger Delay\", \"Memory Acquisition Trigger Duration\", \"Shot Acquisition Trigger Delay\", \"Shot Acquisition Trigger Duration\", \"Acquire Shot\": Value Change;  \"Memory Repetition Period\": Key Down" {
          selector: _ -> [_ _ _]
          dyn-events: _ -> [_ _ _]
          timeout: 100 -> [_ _ _]
          tunnel: [States."Receive Data" ("Enum") States."Send Data" ("Enum") States."Close" ("Enum")] -> w1053
          event #0 {
            n322 = event-data() -> ()  [unwired: 3 out]
          }
          event #1 {
            n323 = event-data() -> ()  [unwired: 5 out]
          }
          event #2 {
            n324 = event-data() -> ()  [unwired: 4 out]
          }
        }
        n325 = local read "Master Stop"() -> (w1055:bool)
        n326 = Select(t=States."Close" ("Enum"), s=w1055, f=w1053) -> (s? t:f=w1052:T12)
      }
      frame #3 {
        w1062 = TRUE ("Stop")
        n327 = disable-structure shown="Enabled" {
          disable-tunnel: w1070 -> [w1074 w1106]
          disable-tunnel: [w1073 w1106] -> w1065
          disable-tunnel: w1064 -> [w1072 w1105]
          disable-tunnel: [w1071 w1105] -> w1063
          frame #0 {
            n328 = xnode "Invoke Method"("FPGA VI Reference In"=w1074, "error in"=w1072) -> ("FPGA VI Reference Out"=w1073:refnum<k20>, "error out"=w1071:errorcluster)
          }
          frame #1 {
          }
        }
        n329 = xnode "Read/Write Control"("FPGA VI Reference In"=w1065, "error in"=w1063, "Stop"=w1062, "WA Stop"=w1062) -> ("FPGA VI Reference Out"=w1069:refnum<k20>, "error out"=w1068:errorcluster)
        "Active" <- FALSE ("Active 2")
      }
      frame #4 {
        w1179 = FALSE ("Show Errors")
        w1259 = FALSE
        w1278 = FALSE ("Show Errors")
        w1284 = FALSE ("Show Errors")
        w1293 = FALSE ("Show Errors")
        # "Chopper Decimation and EIT Sequence Loop"
        n330 = local read "Memory Duration"() -> (w1309:dbl[unit])
        n331 = call "HostConvertTimetoTicks.vi"("Repetition Period"="WA Repetition Period", "Delay (us)"="WA Extra  (DIO0)", "Duration (us)"="WA Extra (DIO0)", "Show Errors"=w1179) -> ("start pulse (tick number)"=w1193:u64, "stop pulse (tick number)"=w1192:u64)  [unwired: 8 in, 2 out]
        n332 = call "HostConvertTimetoTicks.vi"("Repetition Period"="WA Repetition Period", "Delay (us)"="WA Extra 2 (DIO0)", "Duration (us)"="WA Extra 2 (DIO0)", "Show Errors"=w1179) -> ("start pulse (tick number)"=w1186:u64, "stop pulse (tick number)"=w1185:u64)  [unwired: 8 in, 2 out]
        n333 = call "HostConvertTimetoTicks.vi"("Repetition Period"="WA Repetition Period", "Delay (us)"="WA Extra 3 (DIO0)", "Duration (us)"="WA Extra 3 (DIO0)", "Show Errors"=w1179) -> ("start pulse (tick number)"=w1177:u64, "stop pulse (tick number)"=w1176:u64)  [unwired: 8 in, 2 out]
        n334 = call "HostConvertTimetoTicks.vi"("Repetition Period"="WA Repetition Period", "Delay (us)"="WA Extra 4 (DIO0)", "Duration (us)"="WA Extra 4 (DIO0)", "Show Errors"=w1179) -> ("start pulse (tick number)"=w1175:u64, "stop pulse (tick number)"=w1174:u64)  [unwired: 8 in, 2 out]
        n335 = call "HostConvertTimetoTicks.vi"("Repetition Period"="WA Repetition Period", "Delay (us)"="WA Signal Switch (DIO7)", "Duration (us)"="WA Signal Switch (DIO7)", "Show Errors"=w1179) -> ("start pulse (tick number)"=w1190:u64, "stop pulse (tick number)"=w1202:u64)  [unwired: 8 in, 2 out]
        n336 = call "HostConvertTimetoTicks.vi"("Repetition Period"="WA Repetition Period", "Delay (us)"="WA Signal Switch 2  (DIO7)", "Duration (us)"="WA Signal Switch 2 (DIO7)", "Show Errors"=w1179) -> ("start pulse (tick number)"=w1195:u64, "stop pulse (tick number)"=w1194:u64)  [unwired: 8 in, 2 out]
        n337 = call "HostConvertTimetoTicks.vi"("Duration (us)"=w1309, "Show Errors"=w1278) -> ("duration (tick numbers)"=w1310:u64)  [unwired: 10 in, 3 out]
        n338 = call "HostConvertTimetoTicks.vi"("Delay (us)"="Raman Control Delay(DIO5)", "Duration (us)"="Ramand Control Duration (DIO5)", "Show Errors"=w1278) -> ("start pulse (tick number)"=w1288:u64, "stop pulse (tick number)"=w1287:u64)  [unwired: 9 in, 2 out]
        n339 = call "HostConvertTimetoTicks.vi"("Delay (us)"="Raman Signal Delay (DIO6)", "Duration (us)"="Raman Signal Duration (DIO6)", "Show Errors"=w1278) -> ("start pulse (tick number)"=w1290:u64, "stop pulse (tick number)"=w1289:u64)  [unwired: 9 in, 2 out]
        n340 = call "HostConvertTimetoTicks.vi"("Duration (us)"="DLCZ Start", "Show Errors"=w1284) -> ("duration (tick numbers)"=w1298:u64)  [unwired: 10 in, 3 out]
        n341 = call "HostConvertTimetoTicks.vi"("Duration (us)"="DLCZ Stop", "Show Errors"=w1284) -> ("duration (tick numbers)"=w1296:u64)  [unwired: 10 in, 3 out]
        n342 = call "HostConvertTimetoTicks.vi"("Repetition Period"="DLCZ Period", "Duration (us)"="DLCZ Pulse Duration", "Show Errors"=w1293) -> ("duration (tick numbers)"=w1301:u64)  [unwired: 9 in, 3 out]
        n343 = call "HostConvertTimetoTicks.vi"("Repetition Period"="Memory Repetition Period", "Delay (us)"="SQZ AOM Signal Delay (DIO6)", "Duration (us)"="SQZ AOM Signal Duration (DIO6)") -> ("start pulse (tick number)"=w1281:u64, "stop pulse (tick number)"=w1280:u64)  [unwired: 9 in, 2 out]
        n344 = call "HostConvertTimetoTicks.vi"("Duration (us)"="DLCZ Period", "Show Errors"=w1293) -> ("duration (tick numbers)"=w1294:u64)  [unwired: 10 in, 3 out]
        n345 = call "Scale Frequency.vi"("Period"="Memory Repetition Period") -> ("Frequency (scaled)"=w1324:u32)
        n346 = call "HostConvertTimetoTicks.vi"("Repetition Period"="Memory Repetition Period", "Delay (us)"="Control Delay(DIO5/1)", "Duration (us)"="Control Duration (DIO5/1)") -> ("start pulse (tick number)"=w1334:u64, "stop pulse (tick number)"=w1333:u64)  [unwired: 9 in, 2 out]
        n347 = call "HostConvertTimetoTicks.vi"("Repetition Period"="Memory Repetition Period", "Duration (us)"="Trapping (DIO17)", "Show Errors"=FALSE) -> ("duration (tick numbers)"=w1305:u64)  [unwired: 9 in, 3 out]
        n348 = call "HostConvertTimetoTicks.vi"("Repetition Period"="Memory Repetition Period", "Duration (us)"="Pump (DIO19)", "Show Errors"=FALSE) -> ("duration (tick numbers)"=w1304:u64)  [unwired: 9 in, 3 out]
        n349 = call "HostConvertTimetoTicks.vi"("Repetition Period"="Memory Repetition Period", "Duration (us)"="Repump (DIO18)") -> ("duration (tick numbers)"=w1306:u64)  [unwired: 10 in, 3 out]
        n350 = call "HostConvertTimetoTicks.vi"("Repetition Period"="Memory Repetition Period", "Delay (us)"="Coherent Signal Delay (DIO6)", "Duration (us)"="Coherent Signal Duration (DIO6)") -> ("start pulse (tick number)"=w1313:u64, "stop pulse (tick number)"=w1312:u64)  [unwired: 9 in, 2 out]
        n351 = call "HostConvertTimetoTicks.vi"("Repetition Period"="Memory Repetition Period", "Delay (us)"="Opt Density Delay (DIO7)", "Duration (us)"="Opt Density Duration (DIO7)") -> ("start pulse (tick number)"=w1303:u64, "stop pulse (tick number)"=w1302:u64)  [unwired: 9 in, 2 out]
        n352 = call "HostConvertTimetoTicks.vi"("Repetition Period"="WA Repetition Period", "Delay (us)"="WA Control 1 (DIO4)", "Duration (us)"="WA Control 1 (DIO4)", "Show Errors"=w1179) -> ("start pulse (tick number)"=w1250:u64, "stop pulse (tick number)"=w1249:u64)  [unwired: 8 in, 2 out]
        n353 = call "HostConvertTimetoTicks.vi"("Repetition Period"="WA Repetition Period", "Delay (us)"="WA Control 2 (DIO4)", "Duration (us)"="WA Control 2 (DIO4)", "Show Errors"=w1179) -> ("start pulse (tick number)"=w1221:u64, "stop pulse (tick number)"=w1220:u64)  [unwired: 8 in, 2 out]
        n354 = call "HostConvertTimetoTicks.vi"("Repetition Period"="WA Repetition Period", "Delay (us)"="WA Repump (DIO3)", "Duration (us)"="WA Repump (DIO3)", "Show Errors"=w1179) -> ("start pulse (tick number)"=w1222:u64, "stop pulse (tick number)"=w1184:u64)  [unwired: 8 in, 2 out]
        n355 = call "HostConvertTimetoTicks.vi"("Repetition Period"="WA Repetition Period", "Delay (us)"="WA Control Switch 1(DIO6)", "Duration (us)"="WA Control Switch 1 (DIO6)", "Show Errors"=w1179) -> ("start pulse (tick number)"=w1233:u64, "stop pulse (tick number)"=w1232:u64)  [unwired: 8 in, 2 out]
        n356 = call "HostConvertTimetoTicks.vi"("Repetition Period"="WA Repetition Period", "Delay (us)"="WA ControlS 2 (DIO6)", "Duration (us)"="WA ControlS 2 (DIO6)", "Show Errors"=w1179) -> ("start pulse (tick number)"=w1231:u64, "stop pulse (tick number)"=w1230:u64)  [unwired: 8 in, 2 out]
        n357 = call "HostConvertTimetoTicks.vi"("Repetition Period"="WA Repetition Period", "Delay (us)"="WA Pump (DIO2)", "Duration (us)"="WA Pump (DIO2)", "Show Errors"=w1179) -> ("start pulse (tick number)"=w1219:u64, "stop pulse (tick number)"=w1218:u64)  [unwired: 8 in, 2 out]
        n358 = call "HostConvertTimetoTicks.vi"("Repetition Period"="WA Repetition Period", "Delay (us)"="WA Signal (DIO5)", "Duration (us)"="WA Signal (DIO5)", "Show Errors"=w1179) -> ("start pulse (tick number)"=w1227:u64, "stop pulse (tick number)"=w1226:u64)  [unwired: 8 in, 2 out]
        n359 = call "HostConvertTimetoTicks.vi"("Delay (us)"="OD Acquisition Delay", "Show Errors"=w1278) -> ("start pulse (tick number)"=w1277:u64)  [unwired: 10 in, 3 out]
        n360 = call "HostConvertTimetoTicks.vi"("Repetition Period"="Memory Repetition Period", "Delay (us)"="Memory Acquisition Trigger Delay", "Duration (us)"="Memory Acquisition Trigger Duration") -> ("start pulse (tick number)"=w1171:u64, "stop pulse (tick number)"=w1170:u64)  [unwired: 9 in, 2 out]
        n361 = call "HostConvertTimetoTicks.vi"("Repetition Period"="Memory Repetition Period", "Delay (us)"="Shot Acquisition Trigger Delay", "Duration (us)"="Shot Acquisition Trigger Duration") -> ("start pulse (tick number)"=w1167:u64, "stop pulse (tick number)"=w1166:u64)  [unwired: 9 in, 2 out]
        n362 = call "Scale Frequency.vi"("Period"="WA Repetition Period") -> ("Frequency (scaled)"=w1200:u32)
        n363 = call "Scale Frequency.vi"("Period"="SPME Period") -> ("Frequency (scaled)"=w1267:u32)
        n364 = call "HostConvertTimetoTicks.vi"("Duration (us)"="SPME Start", "Show Errors"=w1259) -> ("duration (tick numbers)"=w1264:u64)  [unwired: 10 in, 3 out]
        n365 = call "HostConvertTimetoTicks.vi"("Delay (us)"="SPME Control Delay(DIO5/1)", "Duration (us)"="SPME Control Duration (DIO5/1)", "Show Errors"=w1259) -> ("start pulse (tick number)"=w1274:u64, "stop pulse (tick number)"=w1273:u64)  [unwired: 9 in, 2 out]
        n366 = call "HostConvertTimetoTicks.vi"("Delay (us)"="SPME Signal Gate Delay", "Duration (us)"="SPME Signal Gate Duration", "Show Errors"=w1259) -> ("start pulse (tick number)"=w1254:u64, "stop pulse (tick number)"=w1255:u64)  [unwired: 9 in, 2 out]
        n367 = call "HostConvertTimetoTicks.vi"("Delay (us)"="SPME Signal Delay(DIO5/1)", "Duration (us)"="SPME Signal Duration (DIO5/1)", "Show Errors"=w1259) -> ("start pulse (tick number)"=w1270:u64, "stop pulse (tick number)"=w1269:u64)  [unwired: 9 in, 2 out]
        n368 = call "HostConvertTimetoTicks.vi"("Delay (us)"="SPME Leakage Gate Delay", "Duration (us)"="SPME Leakage Gate Duration", "Show Errors"=w1259) -> ("start pulse (tick number)"=w1256:u64, "stop pulse (tick number)"=w1257:u64)  [unwired: 9 in, 2 out]
        n369 = xnode "Read/Write Control"("FPGA VI Reference In"=w1326, "error in"=w1325, "Control - start"=w1334, "Control - stop"=w1333, "Coherent Signal start"=w1313, "Coherent Signal stop"=w1312, "Trapping Duration"=w1305, "Pump Duration"=w1304, "Repump Duration"=w1306, "Optical Density - start"=w1303, "Optical Density - stop"=w1302, "Repetition Period"=w1324, "DLCZ width"=w1301, "DLCZ Period"=w1294, "DLCZ Start"=w1298, "DLCZ Stop"=w1296, "Output Trigger Sign"="Output  Trigger Sign (DIO13)", "Memory Sequence Duration"=w1310, "Memory Mode"="Memory Mode", "Raman Control - start"=w1288, "Raman Control - stop"=w1287, "Raman Signal - start"=w1290, "Raman Signal - stop"=w1289, "Squeezed AOM Signal stop"=w1280, "Squeezed AOM Signal start"=w1281, "Raman/OD Acquisition Delay"=w1277, "SPME Control - start"=w1274, "SPME Control - stop"=w1273, "SPME Signal start"=w1270, "SPME Signal stop"=w1269, "SPME Period"=w1267, "Num of SPME Pulses per Mem Seq"="Num of SPME Pulses per Mem Seq", "SPME Start"=w1264, "SPME Gate 1 - stop"=w1257, "SPME Gate 1 - start"=w1256, "SPME Gate 2 - stop"=w1255, "SPME Gate 2 - start"=w1254, "Desired Number of Trials"="Desired Number of Trials", "Memory Mode"="Memory", "WA Control Switch Sign"="WA ControlS Sign", "WA Control Switch 1 - start"=w1233, "WA Control Switch 1 - stop"=w1232, "WA Control Switch 2 - start"=w1231, "WA Control Switch 2 - stop"=w1230, "WA Repetition Period"=w1200, "WA Control Sign"="WA Control Sign", "WA Control 1 - start"=w1250, "WA Control 1 - stop"=w1249, "WA Control 2 - start"=w1221, "WA Control 2 - stop"=w1220, "WA Pump Sign"="WA Pump Sign", "WA Pump start"=w1219, "WA Pump stop"=w1218, "WA Repump Sign"="WA Repump Sign", "WA Repump start"=w1222, "WA Repump stop"=w1184, "WA Signal Sign"="WA Signal Sign", "WA Signal start"=w1227, "WA Signal stop"=w1226, "WA Trigger Output Sign"="WA Output  Trigger  Sign (DIO1)", "Coherent Signal Sign"="Coherent Signal Sign", "Raman Control Sign"="Raman Control Sign", "Raman Signal Sign"="Raman Signal Sign", "DLCZ Sign"="DLCZ Sign", "SPME Control Sign"="SPME Control Sign", "SPME Signal Sign"="SPME Signal Sign", "SPME Gate 1 Sign"="SPME Gate1 Sign", "SPME Gate 2 Sign"="SPME Gate2 Sign", "Optical Density Sign"="OD Sign", "Squeezed AOM Control Sign"="SQZ AOM Control Sign", "Squeezed AOM Signal Sign"="SQZ AOM Signal Sign", "Control Sign"="Coherent Control Sign", "WA Signal Switch Sign"="WA Signal Switch Sign", "WA Signal Switch start"=w1190, "WA Signal Switch stop"=w1202, "WA Signal Switch 2 start"=w1195, "WA Signal Switch 2 stop"=w1194, "WA Extra Sign"="WA Extra Sign", "WA Extra start"=w1193, "WA Extra stop"=w1192, "WA Extra start 2"=w1186, "WA Extra stop  2"=w1185, "WA Extra start 3"=w1177, "WA Extra stop  3"=w1176, "WA Extra start 4"=w1175, "WA Extra stop  4"=w1174, "Memory Acquisiton Trigger Delay"=w1171, "Memory Acquisition Trigger Duration"=w1170, "Shot Acquisiton Trigger Delay"=w1167, "Shot Acquisition Trigger Duration"=w1166, "Trigger Shot Aquisition"="Acquire Shot") -> ("FPGA VI Reference Out"=w1327:refnum<k20>, "error out"=w1322:errorcluster, "WA Reset Interval"=→"WA Reset Interval (test)":u64, "WA Active"=→"WA Active":bool)  [unwired: 3 in]
        n370 = Unbundle By Name(w1322) -> ("status"=w1323:bool)
        n371 = Compound Arithmetic op=OR(w1323, "Master Stop") -> (w1258:bool)
        n372 = case shown="False" "Memory" {
          frame #0 {
            # "Do these things when we go into\nalignment mode"
            n373 = property on="Activate Raman Acquisition" class="Bool (strict)"("Val(Sgnl)"=FALSE ("Value (Signaling)")) -> ()  [unwired: 2 in, 2 out]
          }
          frame #1 {
          }
        }
        n374 = Select(t=States."Close" ("Enum"), s=w1258, f=States."Update Graph" ("Enum")) -> (s? t:f=w1319:T12)
      }
      frame #5 {
        n375 = feedback #1() -> (w2806:bool)  [unwired: 1 out]
        "Graphing" <- w2806
        n376 = Not(x=w2806) -> (.not. x?=w2807:bool)
      }
    }
    n377 = Wait (ms)(milliseconds to wait=u32 100) -> ()  [unwired: 1 out]
  }
  n378 = while {
    shift-right: [w2812] -> _
    shift-left: B-Generator_States."Initialize" ("B-Generator States") -> [w2813]
    shift-right: [w2814] -> w54
    shift-left: errorcluster {"status"=FALSE, "code"=0, "source"=""} ("error out") -> [w2809]
    shift-right: [w2815] -> w55
    shift-left: _ -> [w2810]
    stop <- w2811 stop-if-true
    # "B Field Control Signal Generator"
    n379 = case shown="\"Initialize\"" w2813 {
      tunnel: [w2851 w2863 w2870 w2892 w2896] -> w2815
      tunnel: [w2850 w2864 w2869 w2891 w2895] -> w2814
      tunnel: [B-Generator_States."Start Task" ("B-Generator States") B-Generator_States."Check Task" ("B-Generator States") w2868 B-Generator_States."Start Task" ("B-Generator States") B-Generator_States."Stop" ("B-Generator States")] -> w2812
      tunnel: [_ _ _ _ TRUE] -> w2811
      tunnel: w2810 -> [w2849 w2866 w2872 w2894 w2896]
      tunnel: w2809 -> [w2854 w2865 w2871 w2893 w2895]
      frame #0 {
        w2821 = 10171 items=["Rising"=10280, "Falling"=10171] ("edge")
        w2832 = 250000.0
        w2861 = 10178 items=["Finite Samples"=10178, "Continuous Samples"=10123] ("sample mode")
        # "Write Waveform to\nhardware buffer"
        # "Output Pin"
        # "Start Generation on a trigger \nfrom this pin"
        # "Needed so it only writes \nwaveform once per trigger"
        n380 = call-poly <vilib>:"DAQmx Create Virtual Channel.vi"("task in"=w2849, "physical channels"="Output Channel", "error in"=w2854) -> ("task out"=w2856:refnum<k21>, "error out"=w2855:errorcluster)  [unwired: 7 in, 4 out]
        n381 = Select(t="High Voltage (V Hi)", s="Activate B-Field", f=dbl[unit] 0.0 ("Ground")) -> (s? t:f=w2827:dbl[unit])
        n382 = call "B-Field Array Generator.vi"("Final Voltage"="V2", "Initial Voltage"="V1", "Time"="A", "Sample Rate"=w2832) -> ("Voltage Ouputs"=w2852:dbl[])
        n383 = call "B-Field Array Generator.vi"("Final Voltage"="V4", "Initial Voltage"="V3", "Time"="B", "Sample Rate"=w2832) -> ("Voltage Ouputs"=w2853:dbl[])
        n384 = call "B-Field Array Generator.vi"("Final Voltage"=w2827, "Initial Voltage"=w2827, "Time"="Global Delay", "Sample Rate"=w2832) -> ("Voltage Ouputs"=w2831:dbl[])
        n385 = Add(x="Global Delay", y="A") -> (x+y=→"Cut Initiated":dbl[unit])
        n386 = Compound Arithmetic op=ADD("A", "B") -> (→"Memory Duration":dbl[unit])
        n387 = local read "Activate B-Field"() -> (w2823:bool)
        n388 = call-poly <vilib>:"DAQmx Timing.vi"("task/channels in"=w2856, "sample mode"=w2861, "rate"=w2832, "error in"=w2855) -> ("task out"=w2844:refnum<k21>, "error out"=w2859:errorcluster)  [unwired: 3 in, 7 out]
        n389 = Build Array (concatenate)(w2852, w2853) -> (w2830:dbl[])
        n390 = Build Array (concatenate)(w2830, w2831) -> (w2833:dbl[])
        n391 = And(x="Trigger Control", y=w2823) -> (x .and. y?=w2824:bool)
        n392 = Select(t=w2833, s=w2824, f=w2831) -> (s? t:f=w2825:dbl[])
        n393 = call-poly <vilib>:"DAQmx Trigger.vi"("task/channels in"=w2844, "source"="Trigger Source", "edge"=w2821, "error in"=w2859) -> ("task out"=w2843:refnum<k21>, "error out"=w2842:errorcluster)  [unwired: 10 out]
        n394 = Reciprocal(x=w2832) -> (1/x=w2847:dbl)
        n395 = call "B-Field - Bug1 Workaround.vi"("Array 2"=w2825) -> ("Array"=w2829:dbl[])
        "B-Field Control Signal" <- w2829
        n396 = Multiply(x=w2847, y=1000.0) -> (x*y=w2846:dbl)
        n397 = Array Size(array=w2829) -> (size(s)=w2839:i32)
        n398 = property class="DAQmx Timing"(reference=w2843, error in=w2842, "SampQuant.SampPerChan"=w2839) -> (reference out=w2841:refnum<k21>, error out=w2840:errorcluster)
        n399 = Multiply(x=w2846, y=w2839) -> (x*y=w2845:dbl)
        n400 = property on="B-Field Control Signal" class="WFGraph (strict)"("XScale.Multiplier"=w2846, "XScale.Maximum"=w2845) -> ()  [unwired: 2 in, 2 out]
        n401 = call-poly <vilib>:"DAQmx Write.vi"("task/channels in"=w2841, "data"=w2829, "error in"=w2840) -> ("task out"=w2851:refnum<k21>, "error out"=w2850:errorcluster)  [unwired: 1 in, 10 out]
      }
      frame #1 {
        n402 = call <vilib>:"DAQmx Start Task.vi"("task/channels in"=w2866, "error in"=w2865) -> ("task out"=w2863:refnum<k21>, "error out"=w2864:errorcluster)  [unwired: 12 out]
      }
      frame #2 {
        n403 = event shown="[0] Timeout" {
          selector: _ -> [_ _]
          dyn-events: _ -> [_ _]
          timeout: 0 -> [_ _]
          tunnel: [w2880 B-Generator_States."Initialize" ("B-Generator States")] -> w2873
          tunnel: [w2878 _] -> w2870
          tunnel: w2872 -> [w2885 w2888]
          tunnel: w2871 -> [w2884 w2887]
          tunnel: [w2879 w2886] -> w2869
          event #0 {
            n404 = event-data() -> ()  [unwired: 2 out]
            n405 = call <vilib>:"DAQmx Is Task Done.vi"("task/channels in"=w2885, "error in"=w2884) -> ("task out"=w2878:refnum<k21>, "task done?"=w2883:bool, "error out"=w2879:errorcluster)  [unwired: 1 in, 10 out]
            n406 = Select(t=B-Generator_States."Stop Task" ("B-Generator States"), s=w2883, f=B-Generator_States."Check Task" ("B-Generator States")) -> (s? t:f=w2880:T14)
          }
          event #1 {
            n407 = event-data() -> ()  [unwired: 7 out]
            n408 = call <vilib>:"DAQmx Clear Task.vi"("task in"=w2888, "error in"=w2887) -> ("error out"=w2886:errorcluster)  [unwired: 13 out]
          }
        }
        n409 = local read "Master Stop"() -> (w2867:bool)
        n410 = Unbundle By Name(w2869) -> ("status"=w2877:bool)
        n411 = Or(x=w2877, y=w2867) -> (x .or. y?=w2876:bool)
        n412 = Select(t=B-Generator_States."Stop" ("B-Generator States"), s=w2876, f=w2873) -> (s? t:f=w2868:T14)
      }
      frame #3 {
        n413 = call <vilib>:"DAQmx Stop Task.vi"("task/channels in"=w2894, "error in"=w2893) -> ("task out"=w2892:refnum<k21>, "error out"=w2891:errorcluster)  [unwired: 12 out]
      }
      frame #4 {
      }
    }
  }
  n414 = Release Queue(queue=w20, force destroy? (F)=TRUE) -> ()  [unwired: 1 in, 3 out]
  n415 = disable-structure shown="Enabled" {
    frame #0 {
      n416 = local read "Capture"() -> ()  [unwired: 1 in]
    }
    frame #1 {
    }
  }
  n417 = call <vilib>:"DAQmx Clear Task.vi"("task in"=w55, "error in"=w54) -> ("error out"=w56:errorcluster)  [unwired: 13 out]
  n418 = call <vilib>:"Simple Error Handler.vi"("type of dialog (OK msg:1)"=w57, "error in (no error)"=w56) -> ("error out"=w35:errorcluster)  [unwired: 7 out]
  n419 = xnode "Close FPGA VI Reference"("FPGA VI Reference In"=w47, "error in"=w46) -> ("error out"=w48:errorcluster)
  n420 = call <vilib>:"Simple Error Handler.vi"("error in (no error)"=w48) -> ("error out"=w34:errorcluster)  [unwired: 1 in, 7 out]
  n421 = call <vilib>:"Simple Error Handler.vi"("error in (no error)"=w36) -> ("error out"=w32:errorcluster)  [unwired: 1 in, 7 out]
  n422 = Build Array(w35, w34, w33, w32) -> (w31:errorcluster[])
  n423 = call <vilib>:"Merge Errors.vi"("error array in"=w31) -> ("error out"=w50:errorcluster)  [unwired: 3 in, 3 out]
  n424 = case shown="True" TRUE {
    tunnel: w50 -> [w2899 w2903]
    tunnel: [w2899 w2903] -> w49
    frame #0 {
    }
    frame #1 {
      w2901 = FALSE ("Activate Raman Acquisition")
      # "Turn buttons off when\n program is stopped"
      n425 = property on="Activate B-Field" class="Bool (strict)"("Val(Sgnl)"=w2901) -> ()  [unwired: 2 in, 2 out]
      n426 = property on="Acquire Phase" class="Bool (strict)"("Val(Sgnl)"=w2901) -> ()  [unwired: 2 in, 2 out]
      n427 = local write "Master Stop"(FALSE ("Master Stop")) -> ()
      n428 = property on="Acquire Data" class="Bool (strict)"("Val(Sgnl)"=w2901) -> ()  [unwired: 2 in, 2 out]
      n429 = property on="Activate Raman Acquisition" class="Bool (strict)"("Value"=w2901) -> ()  [unwired: 2 in, 2 out]
      n430 = property on="WA Active" class="Bool (strict)"("Value"=FALSE ("WA Active")) -> ()  [unwired: 2 in, 2 out]
    }
  }
  n431 = disable-structure shown="Disabled" {
    disable-tunnel: w49 -> [w2904 _]
    frame #0 {
      n432 = invoke class="VI" method="Default Vals.Reinit All"(error in=w2904) -> ()  [unwired: 2 in, 3 out]
    }
    frame #1 {
    }
  }
